vi "UI_page11.vi"(10 "传递队列输入":refnum<queue>, 11 "notifier":refnum<notifier>) -> ()   [LabVIEW 2012]
uses:
  <vilib>/GPower/VIRegister/Library/Convert/ToSGLArry.vi
  <vilib>/GPower/VIRegister/Library/SubVIs/FindRegisterData.vi
  <vilib>/GPower/VIRegister/Library/SubVIs/ReadSub.vi
  <vilib>/GPower/VIRegister/Library/SubVIs/WriteSub.vi
  <vilib>/GPower/VIRegister/Library/QManager/GetRegisterData.vi
  <vilib>/GPower/Error/Library/SetError.vi
  <vilib>/GPower/Error/Library/FilterCodes.vi
  <vilib>/GPower/Error/Library/Filter/FilterMulti.vi
  <vilib>/GPower/VIRegister/Library/QManager/QManagerAction.vi
  <vilib>/GPower/Error/Library/ErrorType.vi
  <vilib>/GPower/Error/Library/SplitAppended.vi
  <vilib>/GPower/Error/Library/SubVIs/ExplanationToError.vi
  <vilib>/GPower/VIRegister/Library/QManager/GetQName.vi
  <vilib>/GPower/VIRegister/Library/QManager/StartQManager.vi
  <vilib>/Utility/error.llb/Trim Whitespace.vi
  <vilib>/dlg_ctls.llb/Space Constant.vi
  <vilib>/Utility/error.llb/Error Code Database.vi
  <vilib>/GPower/Error/Library/SubVIs/SetStatus.vi
  <vilib>/GPower/Error/Library/AppendErrors.vi
  <vilib>/GPower/Error/Library/Append/AppendSingle.vi
  <vilib>/GPower/VIRegister/VIRegister.lvlib
panel:
  in  "主份温控原状态":bool
  in  "备份复位":bool
  in  "主份加计3断电":bool
  in  "主份加计3加电":bool
  in  "主份陀螺3断电":bool
  in  "主份陀螺3加电":bool
  in  "主份温控关闭":bool
  in  "主份加计2断电":bool
  in  "主份加计1断电":bool
  in  "主份加计2加电":bool
  in  "主份加计1加电":bool
  in  "主份陀螺2断电":bool
  in  "主份陀螺1断电":bool
  in  "主份陀螺2加电":bool
  in  "主份陀螺1加电":bool
  in  "主份温控开启":bool
  in  "备份温控原状态":bool
  in  "主份复位":bool
  in  "备份加计3断电":bool
  in  "备份加计3加电":bool
  in  "备份陀螺3断电":bool
  in  "备份陀螺3加电":bool
  in  "备份温控关闭":bool
  in  "备份加计2断电":bool
  in  "备份加计1断电":bool
  in  "备份加计2加电":bool
  in  "备份加计1加电":bool
  in  "备份陀螺2断电":bool
  in  "备份陀螺1断电":bool
  in  "备份陀螺2加电":bool
  in  "备份陀螺1加电":bool
  in  "备份温控开启":bool
  in  "备份切小量程IF电路":bool
  in  "备份切大量程IF电路":bool
  in  "备份加计全断电":bool
  in  "备份加计全加电":bool
  in  "主份切小量程IF电路":bool
  in  "主份切大量程IF电路":bool
  in  "主份加计全断电":bool
  in  "主份加计全加电":bool
  out "模拟量显示区":string
  out "备份自检状态及船舱标志":string
  out "主份自检状态及船舱标志":string
  out "接收数据统计区域":string
  in  "备份复位远程终端":bool
  in  "备份取消发送器关闭":bool
  in  "备份发送器关闭":bool
  in  "备份发送上一状态字":bool
  in  "主份复位远程终端":bool
  in  "主份取消发送器关闭":bool
  in  "主份发送器关闭":bool
  in  "主份发送上一状态字":bool
  in  "备份RT地址选择":enum32{"RT31", "RT21", "RT9"}(radio)
  in  "主份RT地址选择":enum32{"RT31", "RT21", "RT9"}(radio)
  in  "备份通道选择":enum32{"通道A", "通道B"}(radio)
  in  "主份通道选择":enum32{"通道A", "通道B"}(radio)
  in  "备份自定义周期":u16=10 caption="ms" min=10 max=480
  in  "备份周期设置":enum32{"160ms", "自定义", "480ms", "10ms"}(radio)=enum."10ms"
  in  "主份自定义周期":u16=10 caption="ms" min=10 max=480
  in  "主份周期设置":enum32{"160ms", "自定义", "480ms", "10ms"}(radio)=enum."10ms"
  in  "设置存储信息":bool
  in  "备份存储":bool
  in  "主份存储":bool
  # "主份模式指令"
  # "测量存储区"
  # "备份模式指令"
  # "主份指令"
  # "备份指令"
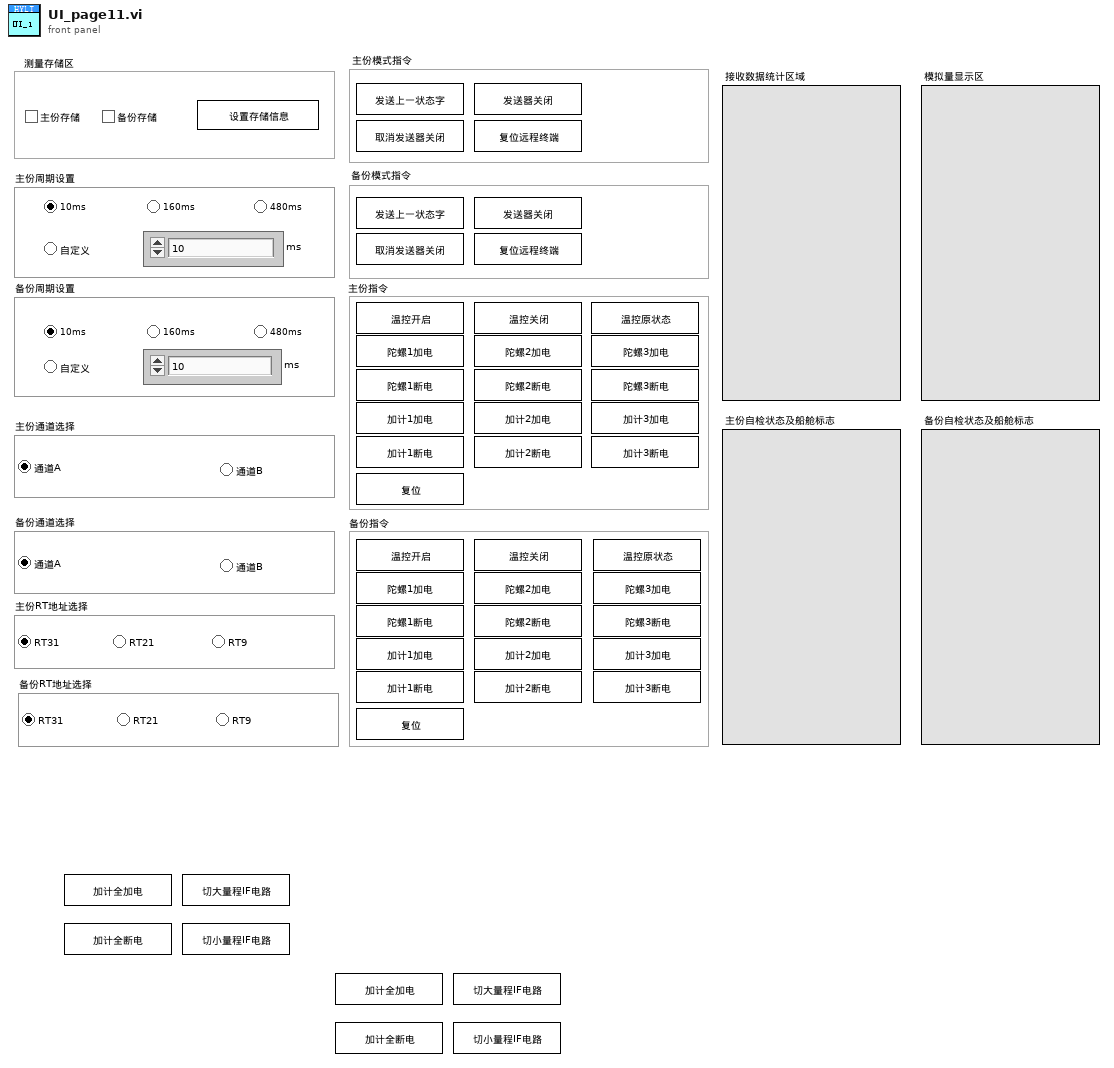
[diagram p1: front panel]
types:
  T1 = cluster{"主份通道选择":enum32{"通道A", "通道B"}, "备份通道选择":enum32{"通道A", "通道B"}}
  T2 = enum32{"invalid app kind", "Development System", "Run Time System", "Student Edition", "Embedded LabVIEW", "Evaluation", "Custom"}
  T3 = enum32{"Invalid", "Standard", "Closed", "Hidden", "Minimized", "Maximized"}
  T4 = cluster{"Core":cluster{"Current VI Reference":refnum<vi>, "Close Panel on Exit?":bool}, "传递队列输入":refnum<queue>, "信息帧":cluster{" 数据帧名称":string, " 数据":string, "备用操作符":bool, "起始地址":i32, "读写标志":i32, "长度":i32}, "主份控制指令":u16, "备份控制指令":u16, "notifier ":refnum<notifier>, "秒计数":i64, "起始时间":i64, "定时控制":bool}
  T5 = cluster{" 数据帧名称":string, " 数据":string, "备用操作符":bool, "起始地址":i32, "读写标志":i32, "长度":i32}
  T6 = cluster{"Current VI Reference":refnum<vi>, "Close Panel on Exit?":bool}
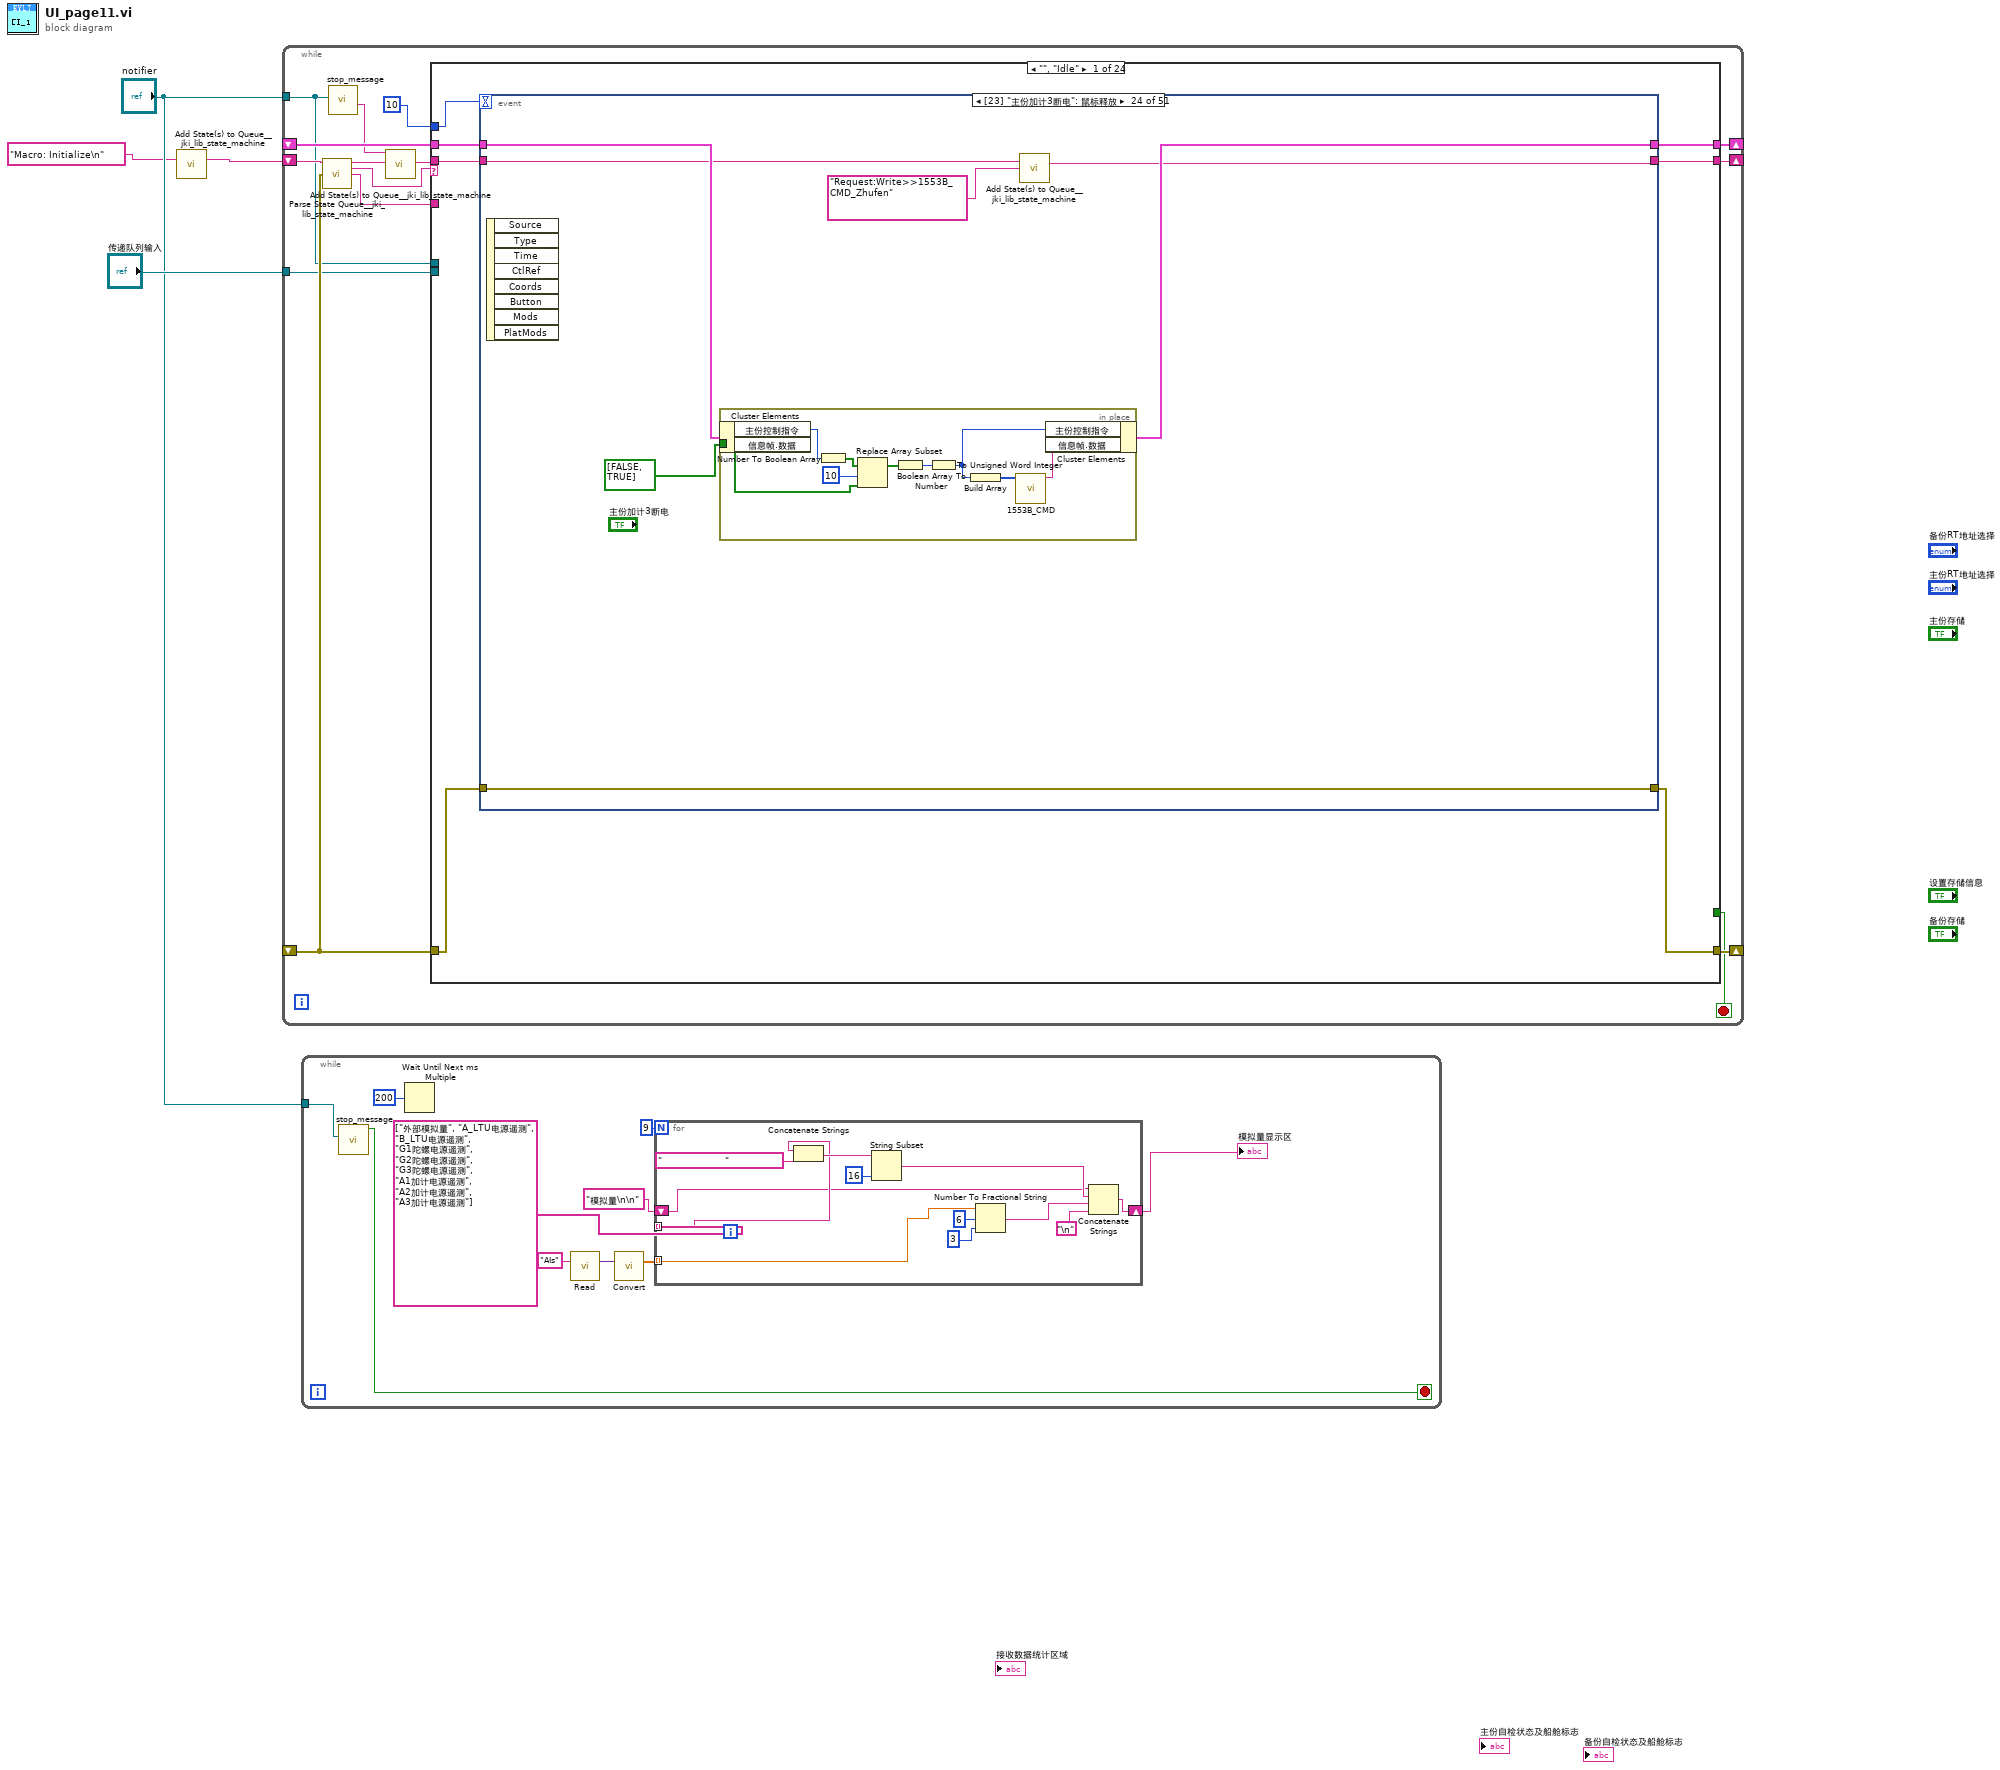
[diagram p0: block diagram]
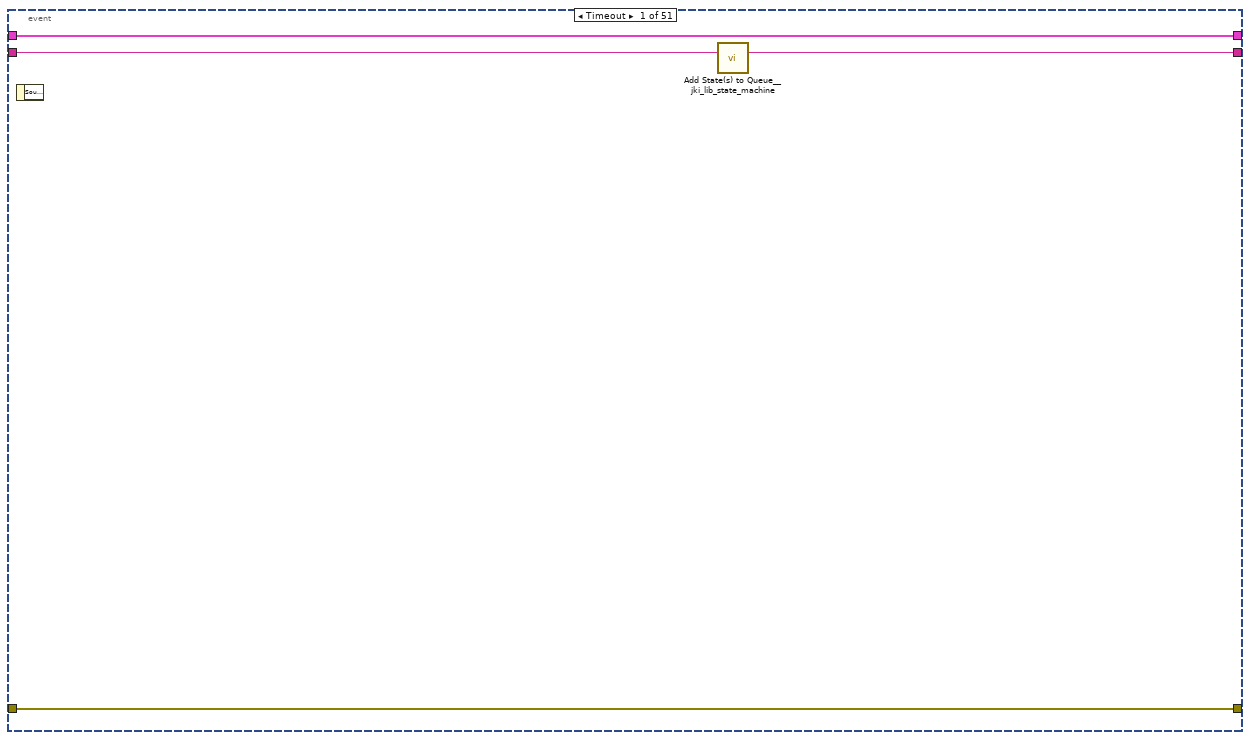
[diagram p2: hidden frame]
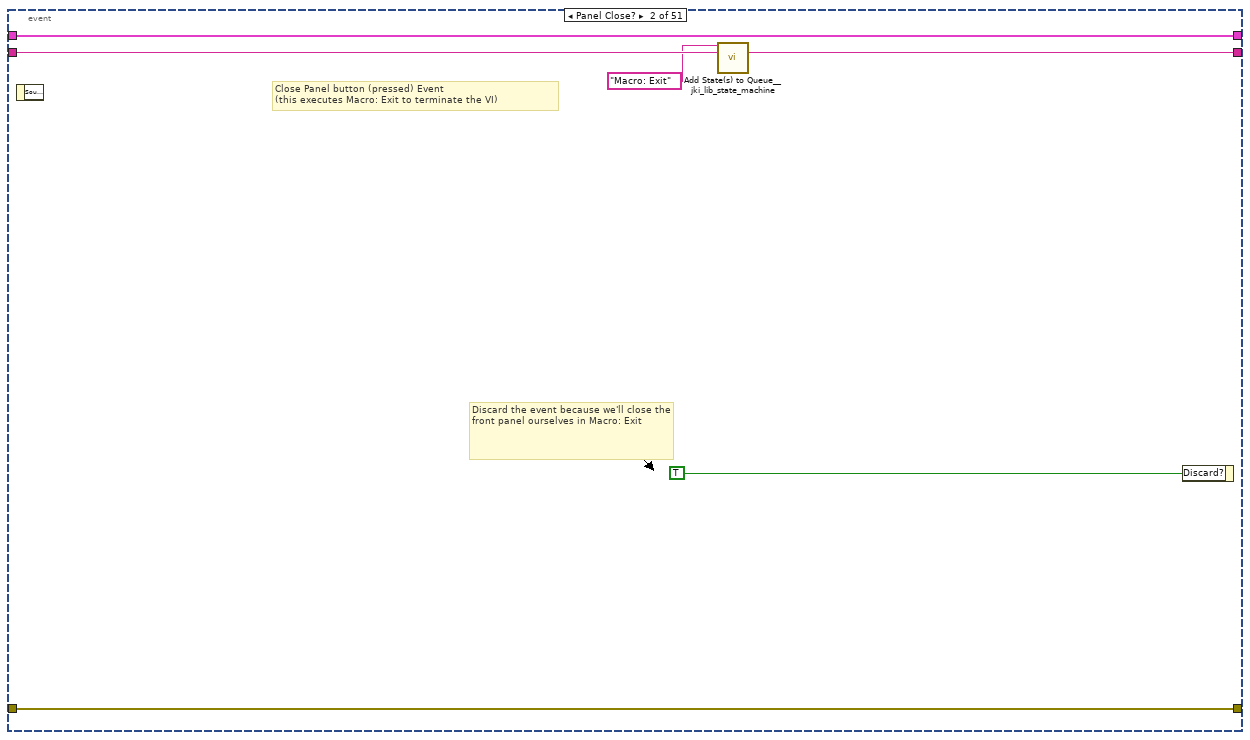
[diagram p3: hidden frame]
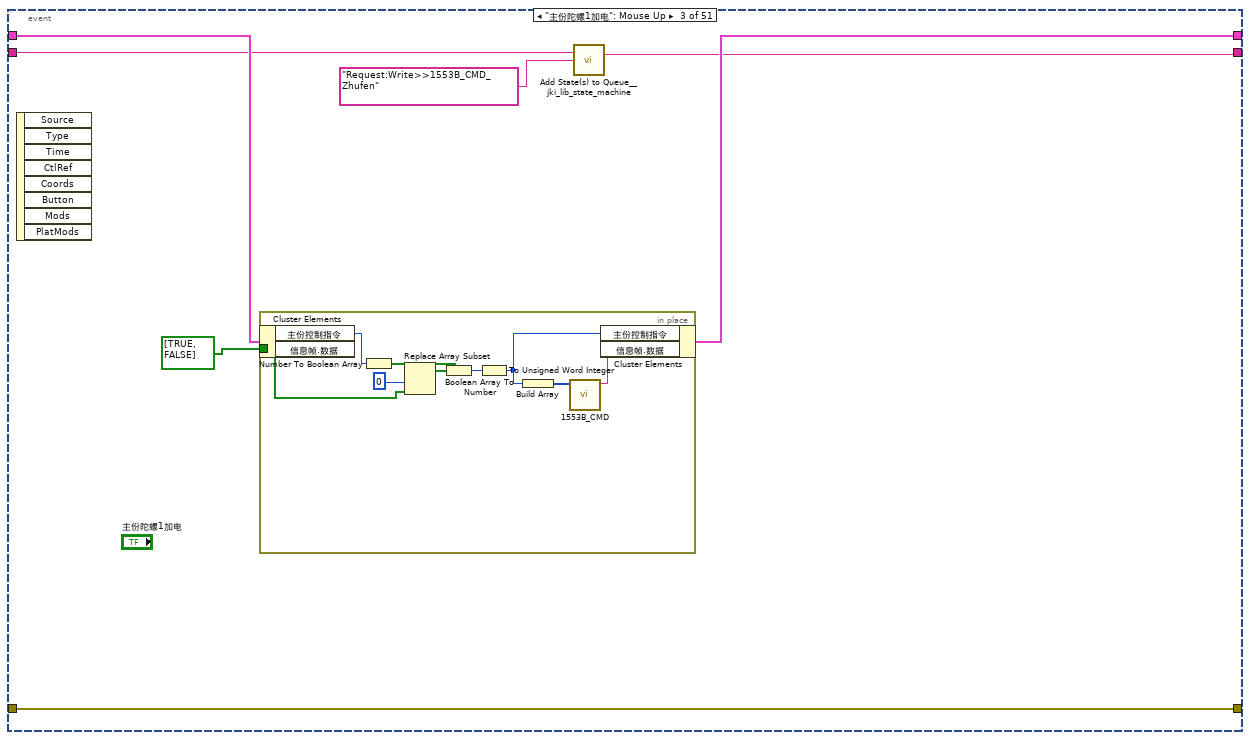
[diagram p4: hidden frame]
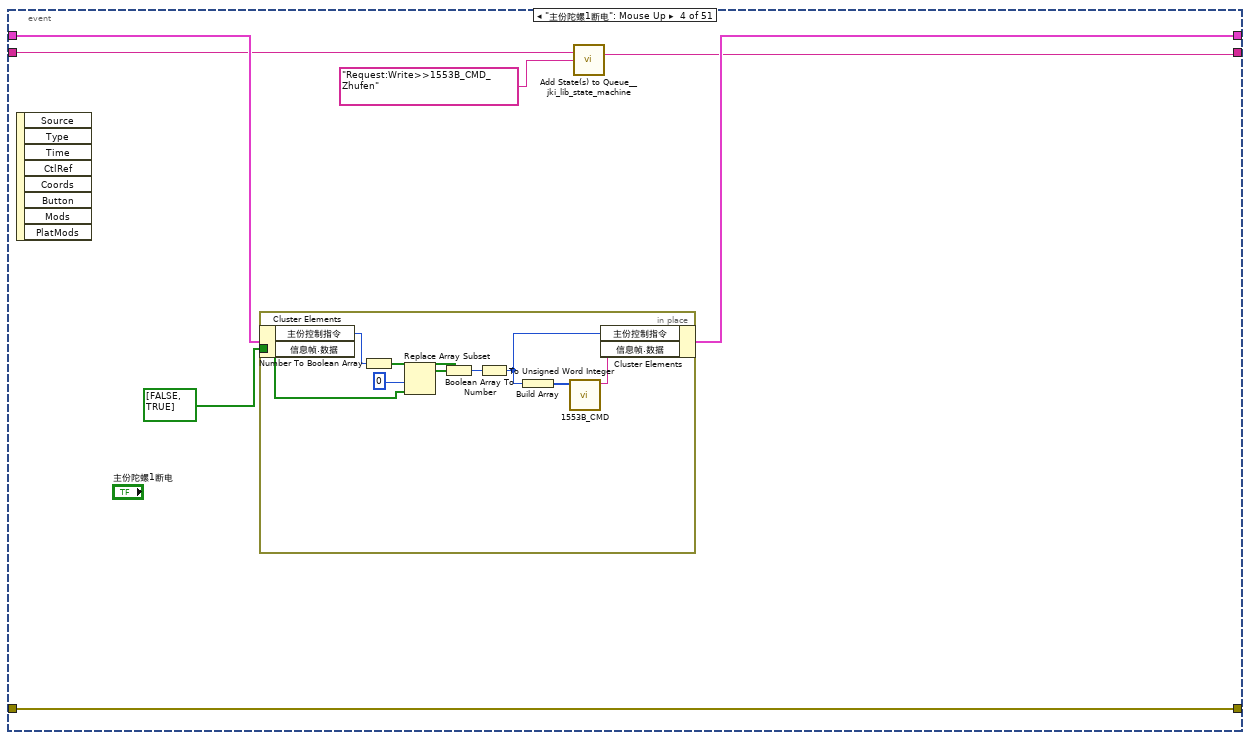
[diagram p5: hidden frame]
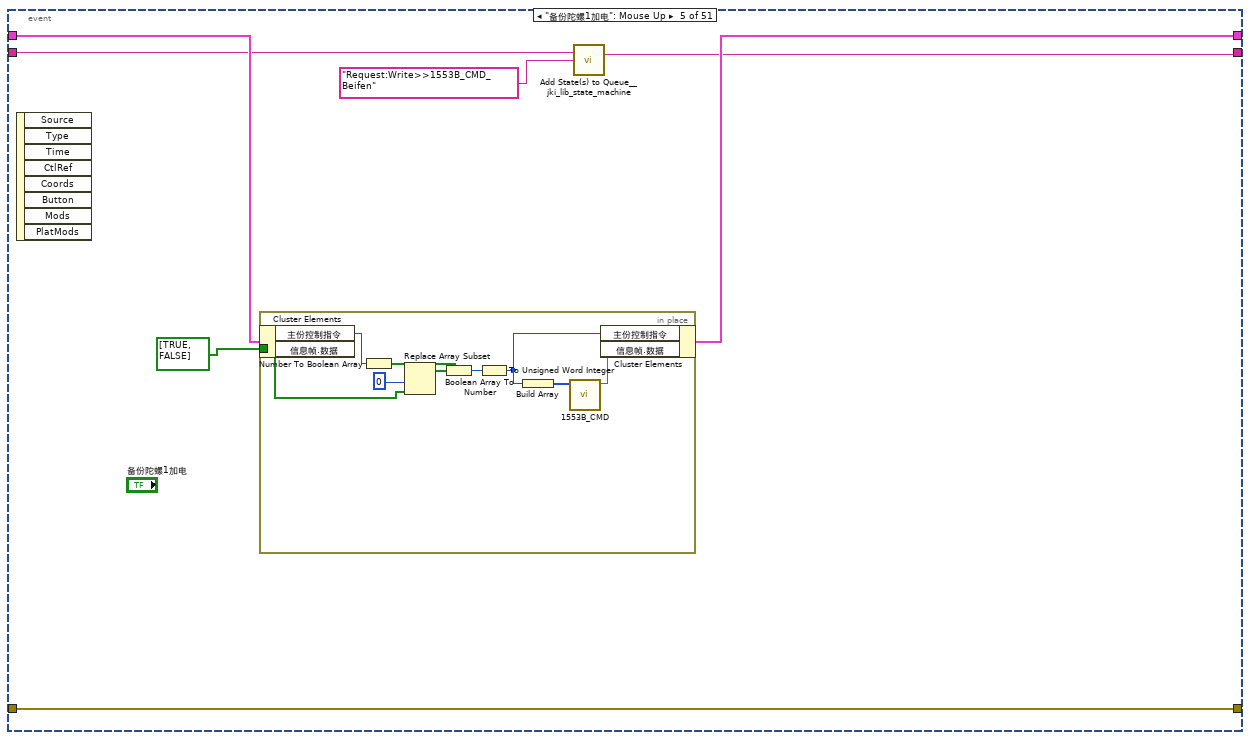
[diagram p6: hidden frame]
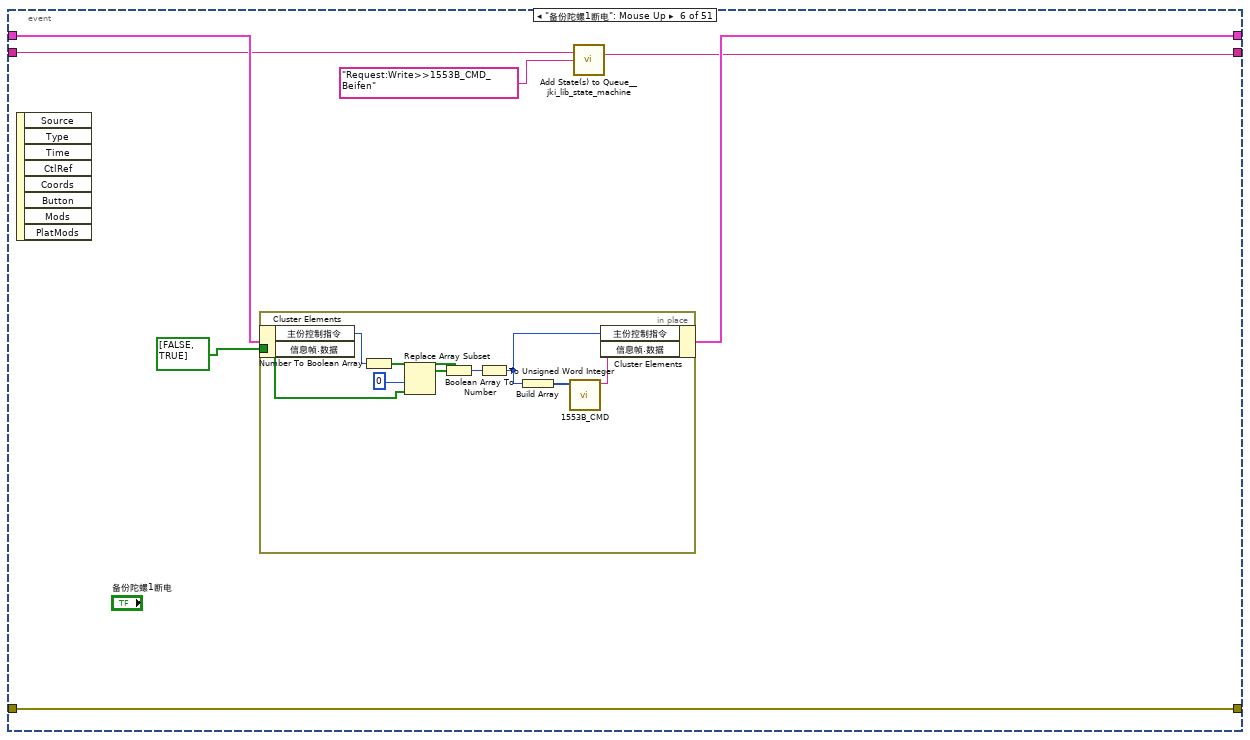
[diagram p7: hidden frame]
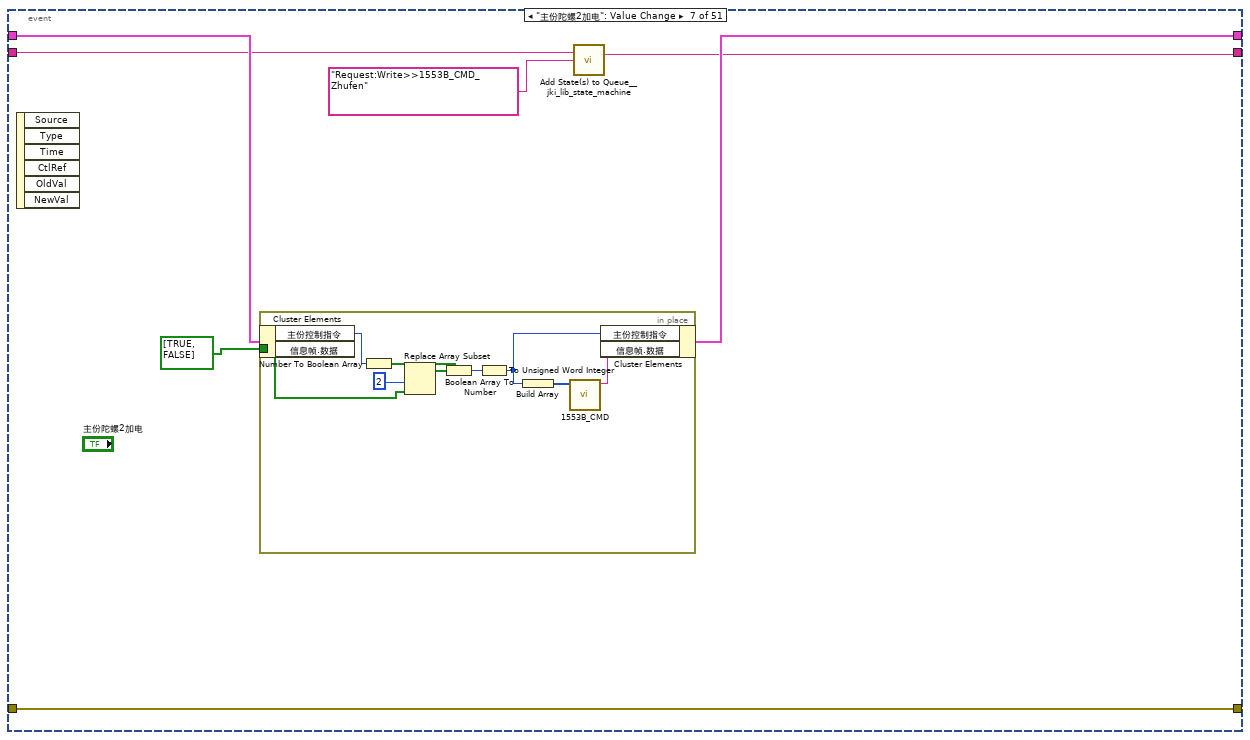
[diagram p8: hidden frame]
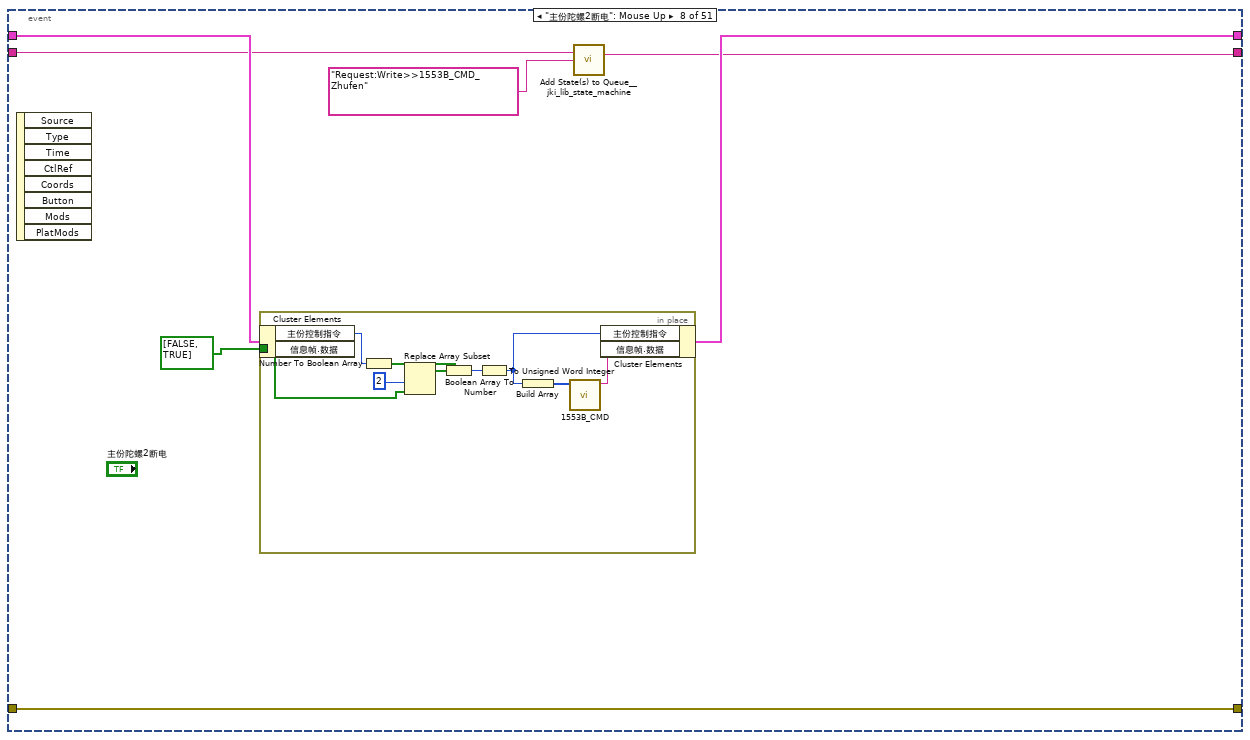
[diagram p9: hidden frame]
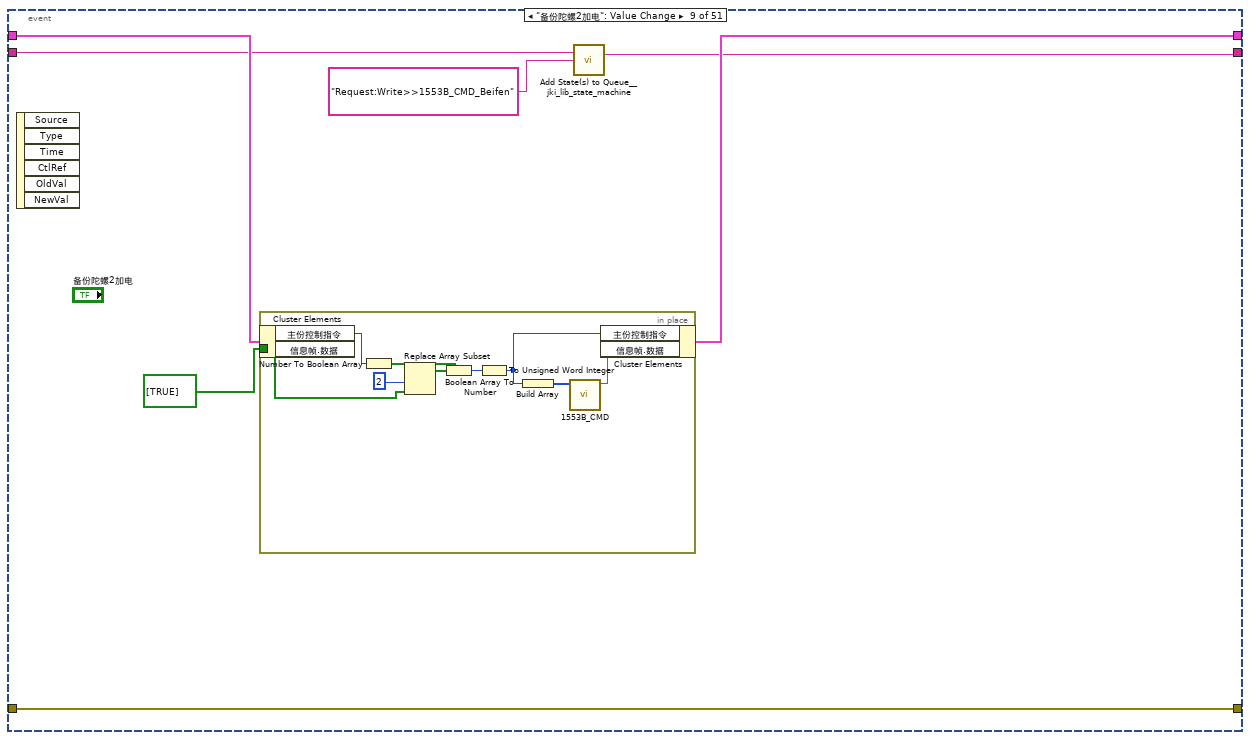
[diagram p10: hidden frame]
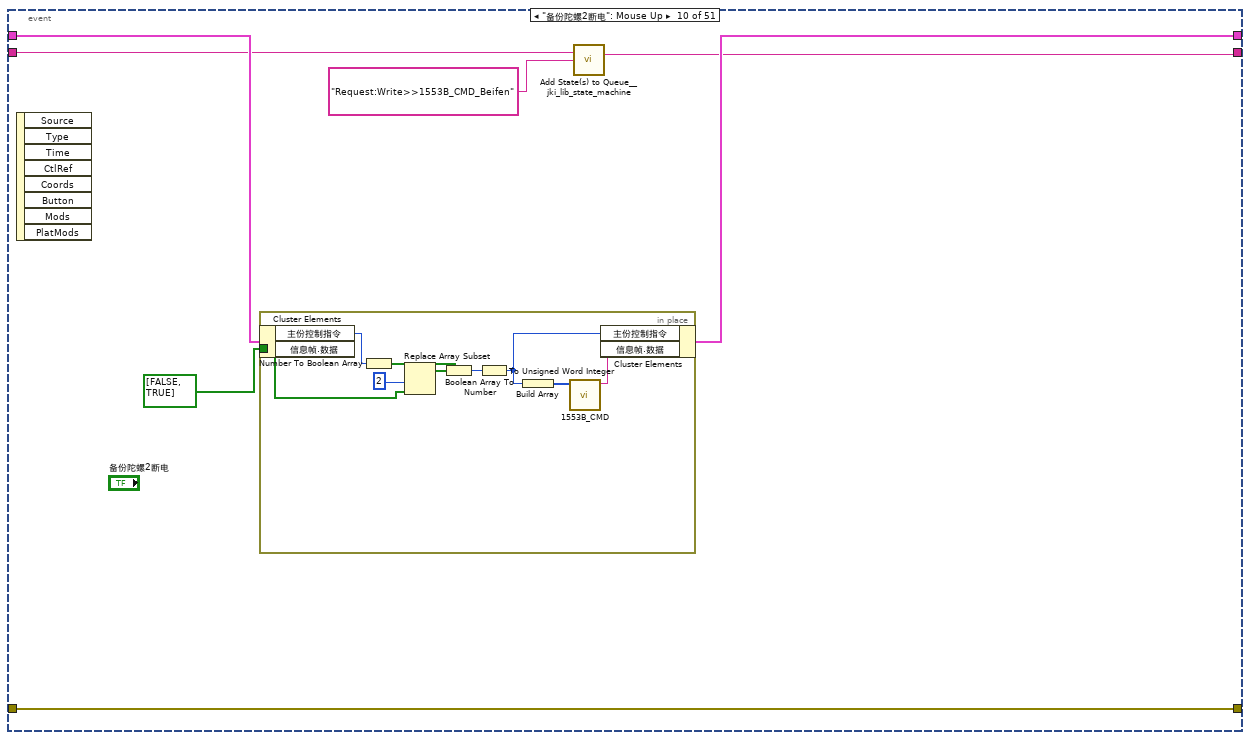
[diagram p11: hidden frame]
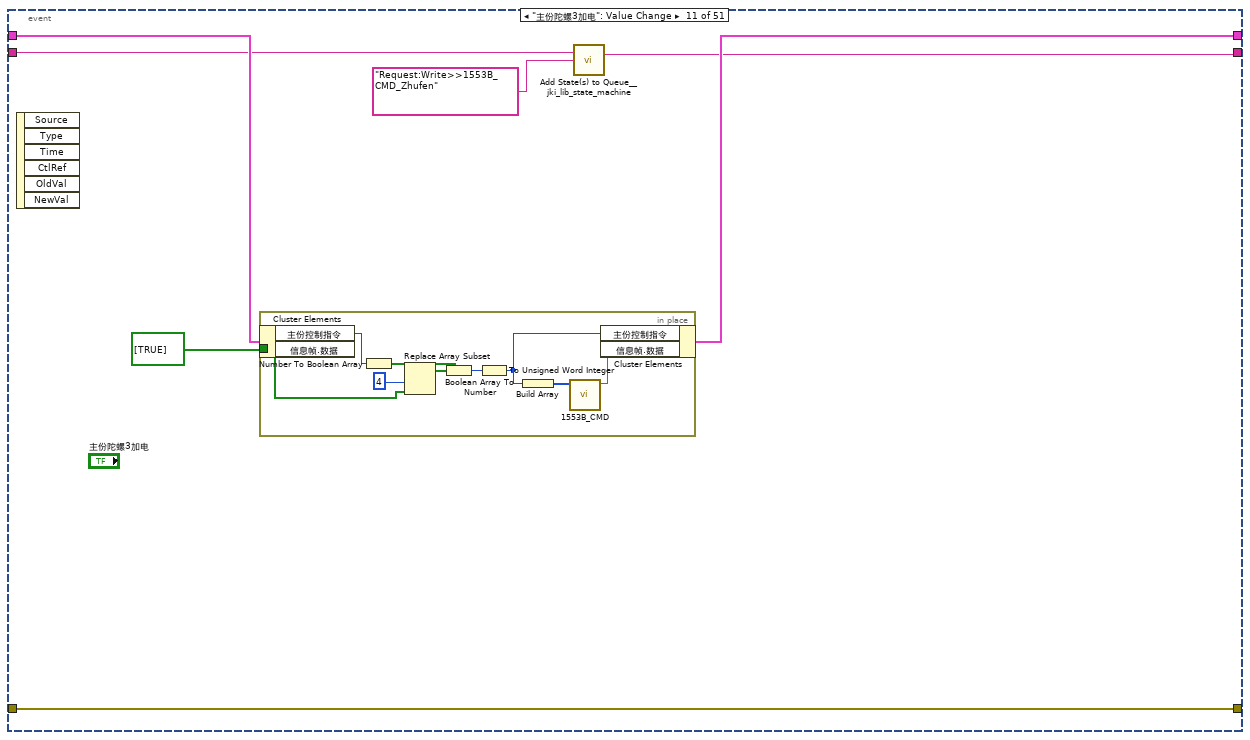
[diagram p12: hidden frame]
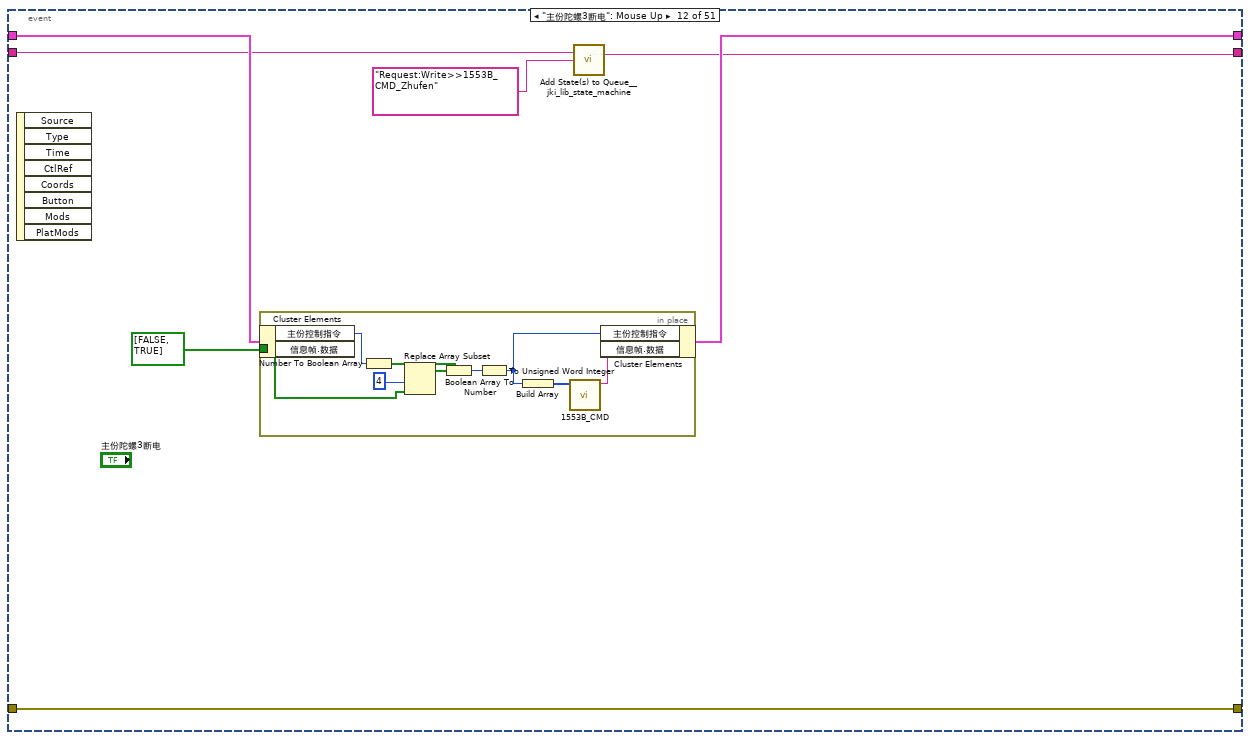
[diagram p13: hidden frame]
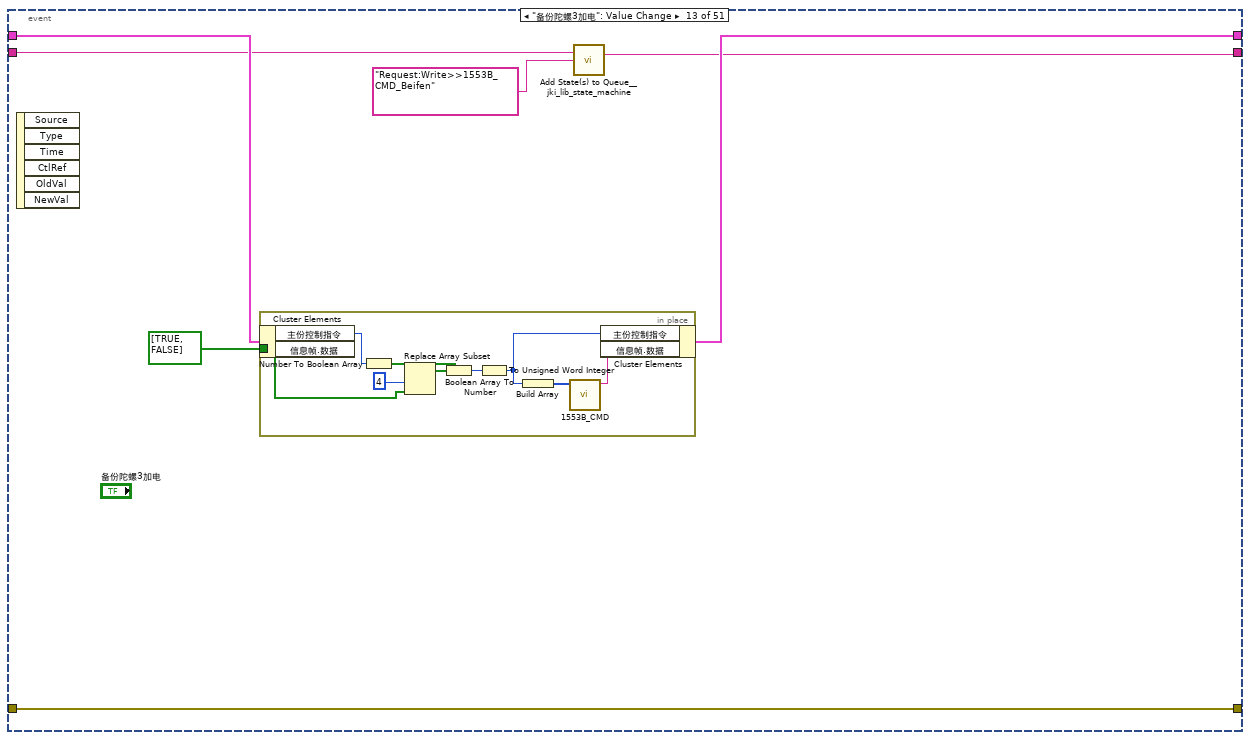
[diagram p14: hidden frame]
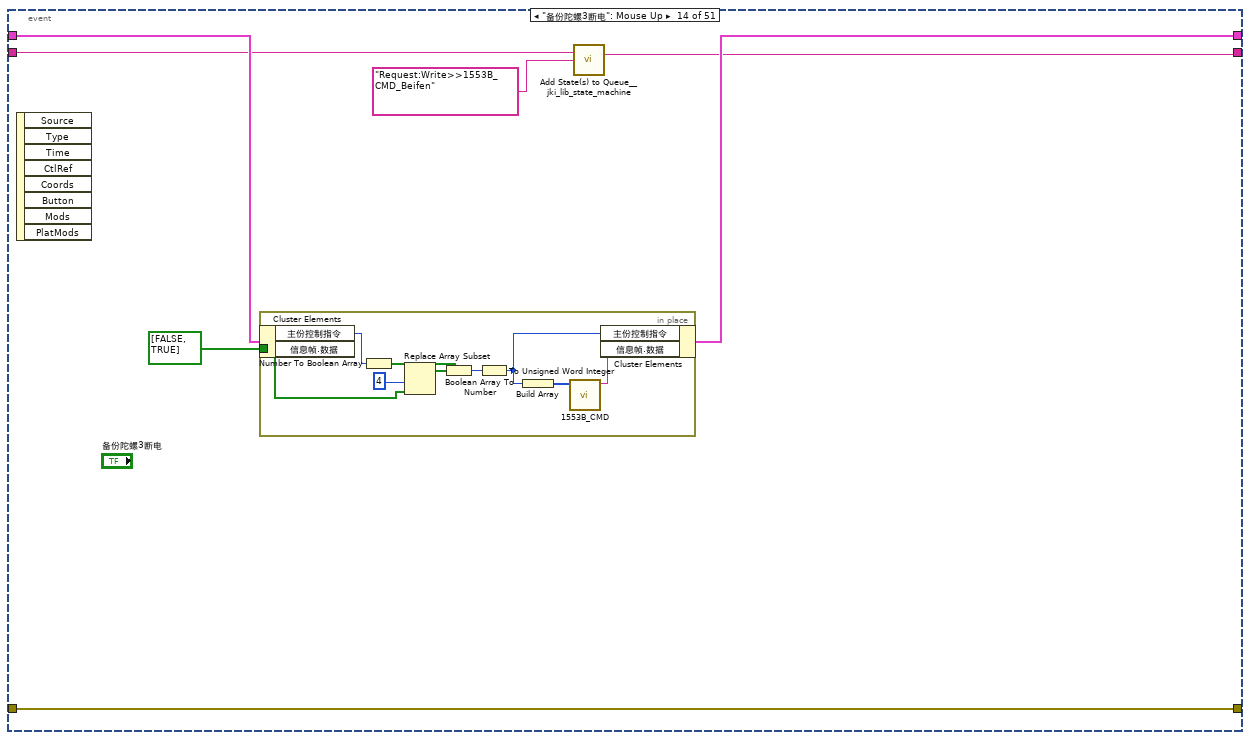
[diagram p15: hidden frame]
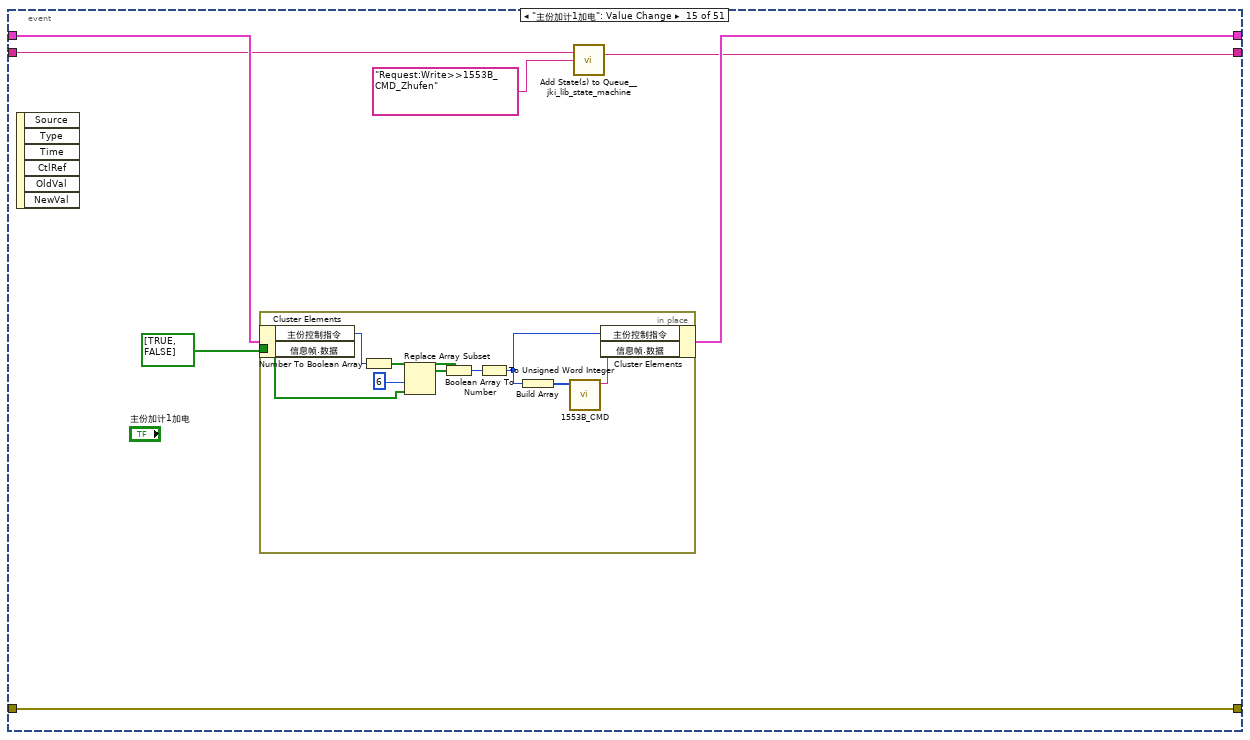
[diagram p16: hidden frame]
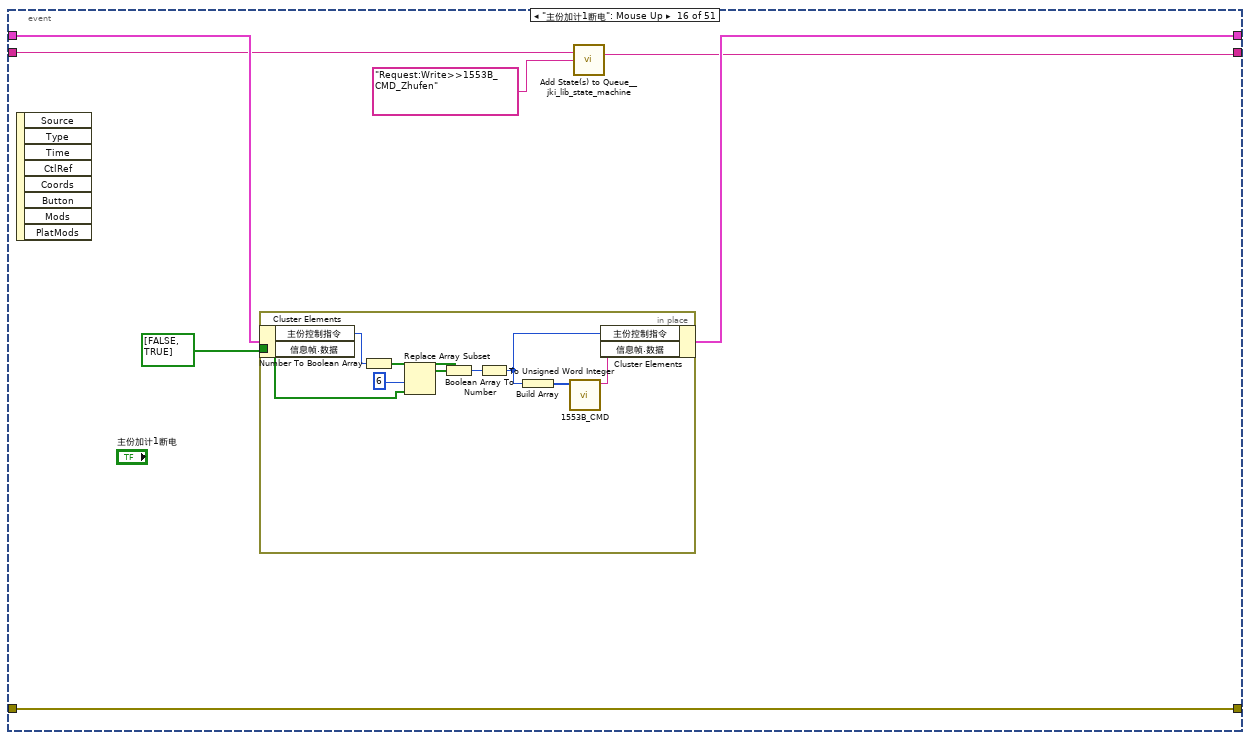
[diagram p17: hidden frame]
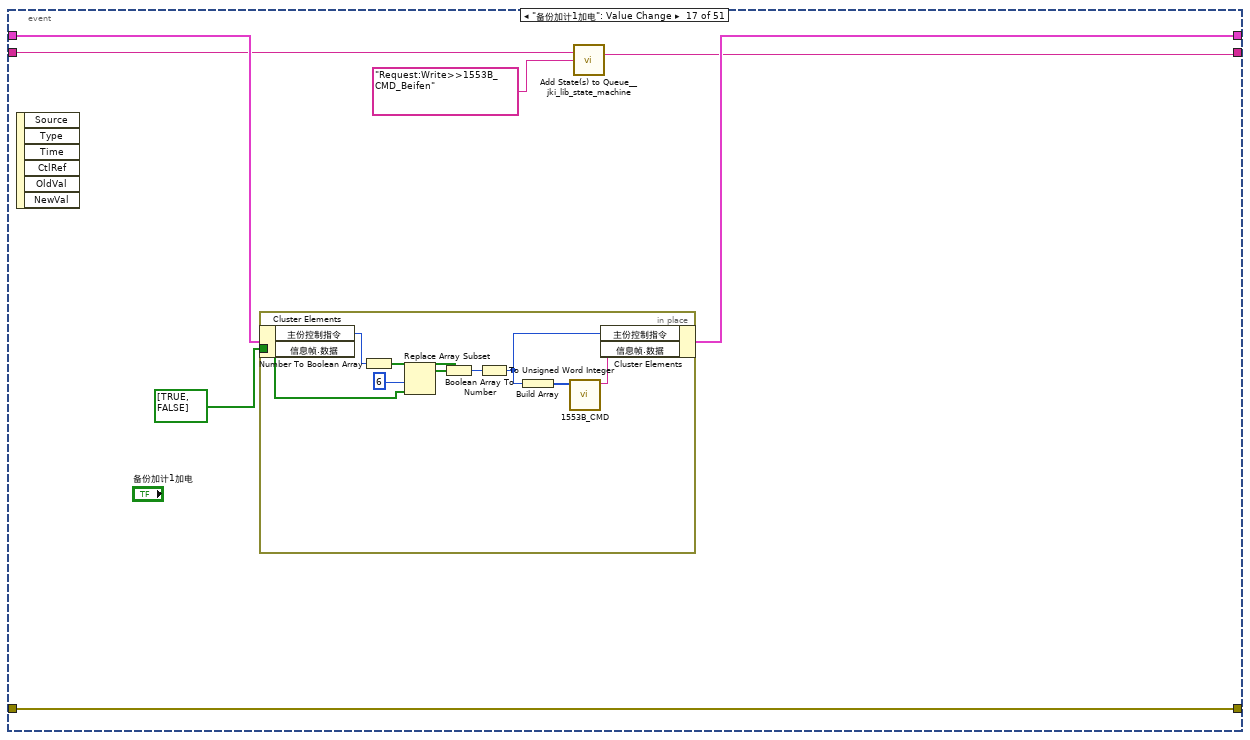
[diagram p18: hidden frame]
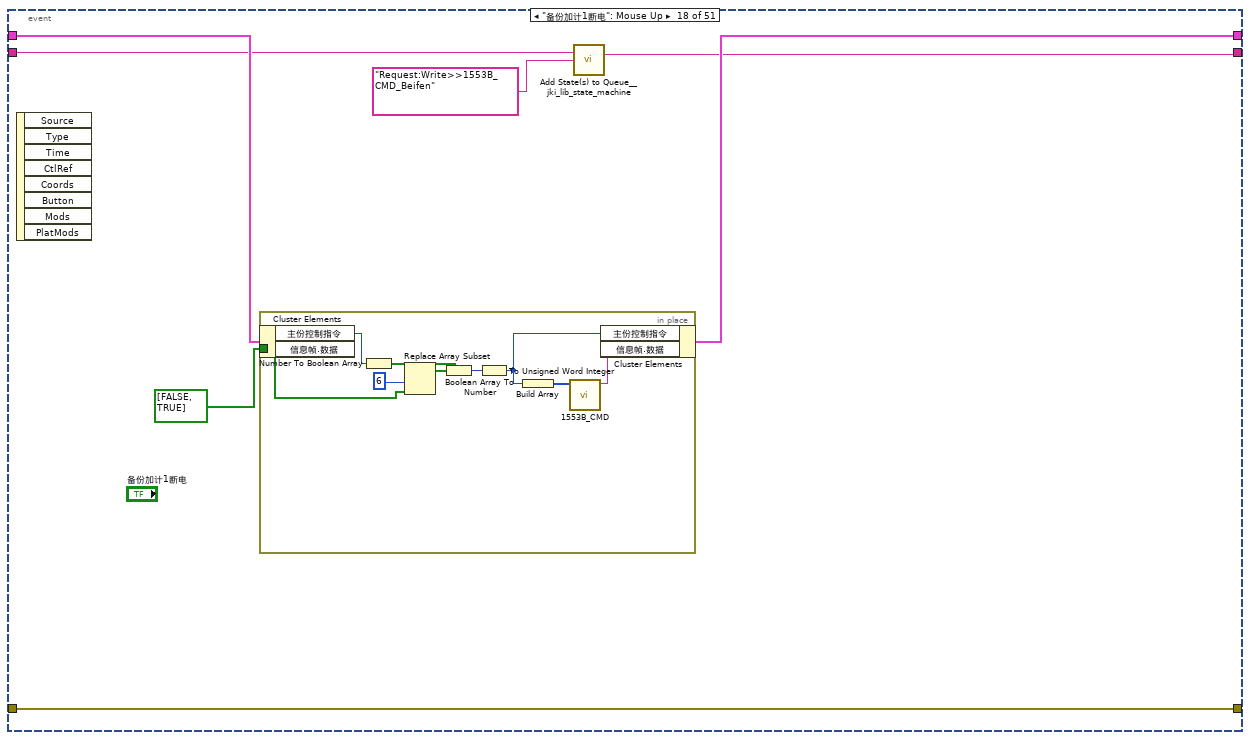
[diagram p19: hidden frame]
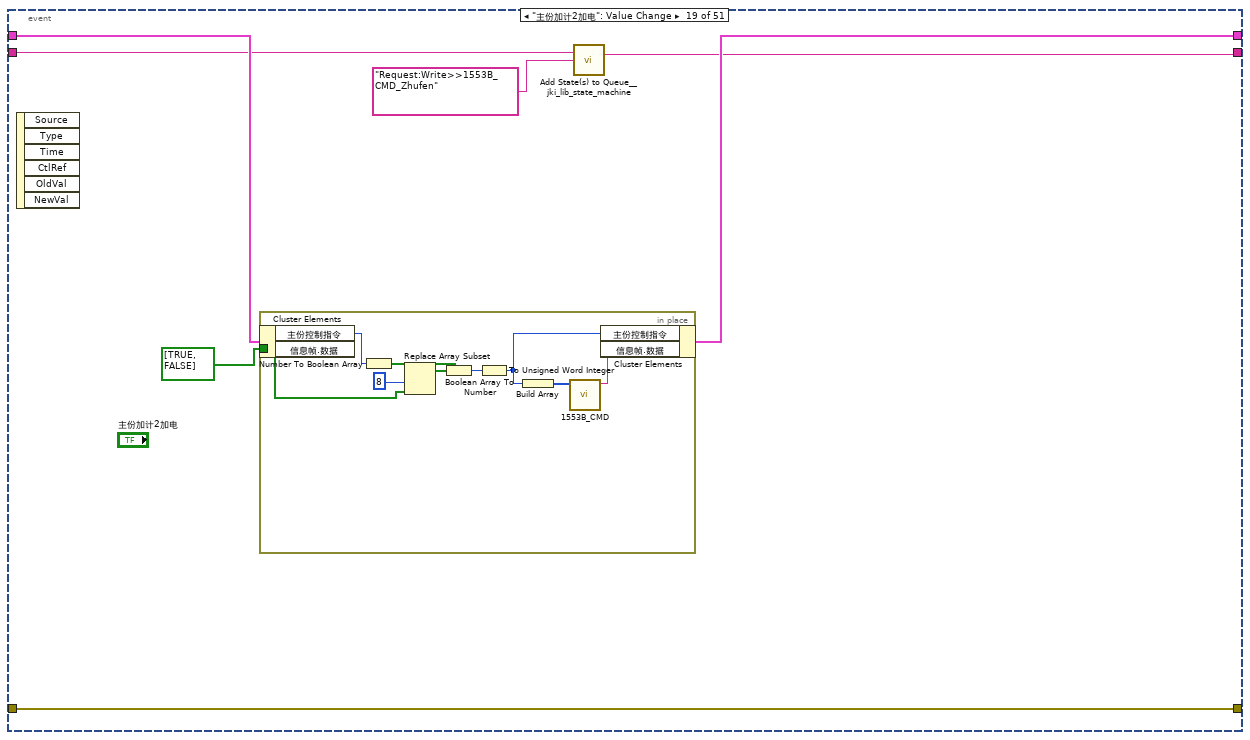
[diagram p20: hidden frame]
diagram:
  n1 = call <vilib>:"Add State(s) to Queue__jki_lib_state_machine.vi"("State(s) in (\"\")"="Macro: Initialize\n") -> ("States Out"=w4:string)  [unwired: 14 in]
  n2 = while "JKI - String-Based Queued State Machine (Basic) v1.0" {
    shift-right: [w13] -> _
    shift-left: _ -> [w12]
    shift-right: [w16] -> _
    shift-left: _ -> [w10]
    shift-right: [w15] -> _
    shift-left: w4 -> [w17]
    tunnel: "notifier" -> [w5]
    tunnel: "传递队列输入" -> [w6]
    stop <- w14 stop-if-true
    n3 = call <vilib>:"Parse State Queue__jki_lib_state_machine.vi"("State Queue"=w17, "Error In (no error)"=w10) -> ("Remaining States"=w9:string, "Current State"=w19:string, "Arguments"=w18:string)  [unwired: 11 in]
    n4 = call "stop_message.vi"("notifier"=w5) -> ("通知"=w8:string)  [unwired: 9 in, 1 out]
    n5 = call <vilib>:"Add State(s) to Queue__jki_lib_state_machine.vi"("State(s) in Front (\"\")"=w8, "State(s) in (\"\")"=w9) -> ("States Out"=w7:string)  [unwired: 13 in]
    n6 = case shown="\"\", \"Idle\"" w19 {
      selector: w19 -> [_ _ w742 _ _ _ _ _ _ _ _ _ _ _ _ _ _ _ _ _ _ _ _ _]
      tunnel: w7 -> [w20 w741 w746 w764 w770 w775 w779 w792 w798 w802 w808 w814 w824 w856 w861 w871 w875 w882 w903 w923 w942 w968 w984 w989]
      tunnel: w18 -> [_ _ _ _ _ _ _ _ _ _ _ w809 w819 _ _ _ _ w876 w897 w917 _ _ _ _]
      tunnel: w12 -> [w25 w738 w744 w755 w767 w773 w776 _ w793 w799 w806 w812 w820 w853 w858 w868 w872 w880 w901 w921 w940 w966 w981 w986]
      tunnel: [w24 w739 w748 w761 errorcluster {"status"=FALSE, "code"=0, "source"=""} ("error out") w772 w777 w789 w794 w800 w805 w810 w821 w854 w859 w869 w873 w878 w899 w919 w938 w964 w982 w987] -> w16
      tunnel: w10 -> [w23 w739 w747 w761 w766 w772 w777 w789 w795 w800 w805 w811 w822 w854 w859 w869 w873 w879 w900 w920 w939 w965 w982 w987]
      tunnel: [w26 w740 w745 w763 w769 w774 w778 w791 w797 w801 w807 w813 w823 w855 w860 w870 w874 w881 w902 w922 w941 w967 w983 w988] -> w15
      tunnel: [_ _ _ _ _ TRUE _ _ _ _ _ _ _ _ _ _ _ _ _ _ _ _ _ _] -> w14
      tunnel: [w22 w738 w744 w762 w767 w773 w776 w790 w793 w799 w806 w812 w820 w853 w858 w868 w872 w877 w898 w918 w937 w963 w981 w986] -> w13
      tunnel: 10 ("Timeout") -> [w21 _ _ _ _ _ _ _ _ _ _ _ _ _ _ _ _ _ _ _ _ _ _ _]
      tunnel: w6 -> [_ _ _ _ _ _ _ w786 _ _ _ _ _ _ _ _ _ _ _ _ _ _ _ _]
      tunnel: w5 -> [_ _ _ _ _ _ _ w783 _ _ _ _ _ _ _ _ _ _ _ _ _ _ _ _]
      frame "", "Idle" {
        n7 = event shown="[23] \"主份加计3断电\": 鼠标释放" {
          selector: _ -> [_ _ _ _ _ _ _ _ _ _ _ _ _ _ _ _ _ _ _ _ _ _ _ _ _ _ _ _ _ _ _ _ _ _ _ _ _ _ _ _ _ _ _ _ _ _ _ _ _ _ _]
          dyn-events: _ -> [_ _ _ _ _ _ _ _ _ _ _ _ _ _ _ _ _ _ _ _ _ _ _ _ _ _ _ _ _ _ _ _ _ _ _ _ _ _ _ _ _ _ _ _ _ _ _ _ _ _ _]
          timeout: w21 -> [_ _ _ _ _ _ _ _ _ _ _ _ _ _ _ _ _ _ _ _ _ _ _ _ _ _ _ _ _ _ _ _ _ _ _ _ _ _ _ _ _ _ _ _ _ _ _ _ _ _ _]
          tunnel: w20 -> [w30 w36 w41 w57 w73 w89 w105 w121 w137 w153 w169 w185 w201 w217 w233 w249 w265 w281 w297 w313 w329 w345 w361 w377 w393 w409 w430 w446 w455 w464 w473 w482 w491 w500 w509 w516 w543 w564 w585 w605 w616 w630 w651 w669 w678 w687 w696 w705 w714 w723 w732]
          tunnel: [w29 w35 w39 w55 w71 w87 w103 w119 w135 w151 w167 w183 w199 w215 w231 w247 w263 w279 w295 w311 w327 w343 w359 w375 w391 w407 w428 w444 w453 w462 w471 w480 w489 w498 w507 w515 w542 w563 w584 w604 w614 w628 w649 w667 w676 w685 w694 w703 w712 w721 w730] -> w26
          tunnel: w25 -> [w27 w33 w43 w59 w75 w91 w107 w123 w139 w155 w171 w187 w203 w219 w235 w251 w267 w283 w299 w315 w331 w347 w363 w379 w395 w411 w422 w448 w457 w466 w475 w484 w493 w502 w511 w518 w546 w566 w587 w602 w618 w632 w653 w671 w680 w689 w698 w707 w716 w725 w734]
          tunnel: [w28 w34 w38 w54 w70 w86 w102 w118 w134 w150 w166 w182 w198 w214 w230 w246 w262 w278 w294 w310 w326 w342 w358 w374 w390 w406 w427 w443 w452 w461 w470 w479 w488 w497 w506 w514 w541 w555 w576 w597 w613 w627 w648 w666 w675 w684 w693 w702 w711 w720 w729] -> w24
          tunnel: w23 -> [w28 w34 w38 w54 w70 w86 w102 w118 w134 w150 w166 w182 w198 w214 w230 w246 w262 w278 w294 w310 w326 w342 w358 w374 w390 w406 w427 w443 w452 w461 w470 w479 w488 w497 w506 w514 w541 w559 w579 w598 w613 w627 w648 w666 w675 w684 w693 w702 w711 w720 w729]
          tunnel: [w27 w33 w42 w58 w74 w90 w106 w122 w138 w154 w170 w186 w202 w218 w234 w250 w266 w282 w298 w314 w330 w346 w362 w378 w394 w410 w421 w447 w456 w465 w474 w483 w492 w501 w510 w517 w544 w565 w586 w601 w617 w631 w652 w670 w679 w688 w697 w706 w715 w724 w733] -> w22
          event Timeout {
            n8 = event-data() -> ()  [unwired: 1 in, 1 out]
            n9 = call <vilib>:"Add State(s) to Queue__jki_lib_state_machine.vi"("State(s) in (\"\")"=w30) -> ("States Out"=w29:string)  [unwired: 14 in]
          }
          event Panel Close? {
            # "Discard the event because we'll close the front panel ourselves in Macro: Exit"
            # "Close Panel button (pressed) Event\n(this executes Macro: Exit to terminate the VI)"
            n10 = event-data() -> ()  [unwired: 1 in, 1 out]
            n11 = call <vilib>:"Add State(s) to Queue__jki_lib_state_machine.vi"("State(s) in Front (\"\")"="Macro: Exit", "State(s) in (\"\")"=w36) -> ("States Out"=w35:string)  [unwired: 13 in]
            n12 = event-data("Discard?"=TRUE) -> ()  [unwired: 1 in, 1 out]
          }
          event "主份陀螺1加电": Mouse Up {
            n13 = event-data() -> ()  [unwired: 1 in, 8 out]
            n14 = in-place {
              in-place-border: bool[] [TRUE, FALSE] -> [w47]
              n15 = in-place-cluster #1(w43) -> ("主份控制指令"=w52:u16)  [unwired: 1 out]
              n16 = Number To Boolean Array(number=w52) -> (Boolean array=w50:bool[])
              n17 = Replace Array Subset(array=w50, new element=w47, index=0 ("索引")) -> (w48:bool[])
              n18 = Boolean Array To Number(Boolean array=w48) -> (number=w51:u32)
              n19 = To Unsigned Word Integer(number=w51) -> (unsigned 16bit integer=w46:u16)
              n20 = Build Array(w46) -> (w45:u16[])
              n21 = call "1553B_CMD.vi"("数据字数组"=w45) -> ("1553B指令"=w44:string)  [unwired: 10 in]
              n22 = in-place-cluster #1("主份控制指令"=w46, "信息帧.数据"=w44) -> (w42:T4)
            }
            n23 = call <vilib>:"Add State(s) to Queue__jki_lib_state_machine.vi"("State(s) in (\"\")"=w41, "State(s) at Back (\"\")"="Request:Write>>1553B_CMD_Zhufen") -> ("States Out"=w39:string)  [unwired: 13 in]
          }
          event "主份陀螺1断电": Mouse Up {
            n24 = event-data() -> ()  [unwired: 1 in, 8 out]
            n25 = in-place {
              in-place-border: bool[] [FALSE, TRUE] -> [w63]
              n26 = in-place-cluster #2(w59) -> ("主份控制指令"=w68:u16)  [unwired: 1 out]
              n27 = Number To Boolean Array(number=w68) -> (Boolean array=w66:bool[])
              n28 = Replace Array Subset(array=w66, new element=w63, index=0 ("索引")) -> (w64:bool[])
              n29 = Boolean Array To Number(Boolean array=w64) -> (number=w67:u32)
              n30 = To Unsigned Word Integer(number=w67) -> (unsigned 16bit integer=w62:u16)
              n31 = Build Array(w62) -> (w61:u16[])
              n32 = call "1553B_CMD.vi"("数据字数组"=w61) -> ("1553B指令"=w60:string)  [unwired: 10 in]
              n33 = in-place-cluster #2("主份控制指令"=w62, "信息帧.数据"=w60) -> (w58:T4)
            }
            n34 = call <vilib>:"Add State(s) to Queue__jki_lib_state_machine.vi"("State(s) in (\"\")"=w57, "State(s) at Back (\"\")"="Request:Write>>1553B_CMD_Zhufen") -> ("States Out"=w55:string)  [unwired: 13 in]
          }
          event "备份陀螺1加电": Mouse Up {
            n35 = event-data() -> ()  [unwired: 1 in, 8 out]
            n36 = in-place {
              in-place-border: bool[] [TRUE, FALSE] -> [w79]
              n37 = in-place-cluster #3(w75) -> ("主份控制指令"=w84:u16)  [unwired: 1 out]
              n38 = Number To Boolean Array(number=w84) -> (Boolean array=w82:bool[])
              n39 = Replace Array Subset(array=w82, new element=w79, index=0 ("索引")) -> (w80:bool[])
              n40 = Boolean Array To Number(Boolean array=w80) -> (number=w83:u32)
              n41 = To Unsigned Word Integer(number=w83) -> (unsigned 16bit integer=w78:u16)
              n42 = Build Array(w78) -> (w77:u16[])
              n43 = call "1553B_CMD.vi"("数据字数组"=w77) -> ("1553B指令"=w76:string)  [unwired: 10 in]
              n44 = in-place-cluster #3("主份控制指令"=w78, "信息帧.数据"=w76) -> (w74:T4)
            }
            n45 = call <vilib>:"Add State(s) to Queue__jki_lib_state_machine.vi"("State(s) in (\"\")"=w73, "State(s) at Back (\"\")"="Request:Write>>1553B_CMD_Beifen") -> ("States Out"=w71:string)  [unwired: 13 in]
          }
          event "备份陀螺1断电": Mouse Up {
            n46 = event-data() -> ()  [unwired: 1 in, 8 out]
            n47 = in-place {
              in-place-border: bool[] [FALSE, TRUE] -> [w95]
              n48 = in-place-cluster #4(w91) -> ("主份控制指令"=w100:u16)  [unwired: 1 out]
              n49 = Number To Boolean Array(number=w100) -> (Boolean array=w98:bool[])
              n50 = Replace Array Subset(array=w98, new element=w95, index=0 ("索引")) -> (w96:bool[])
              n51 = Boolean Array To Number(Boolean array=w96) -> (number=w99:u32)
              n52 = To Unsigned Word Integer(number=w99) -> (unsigned 16bit integer=w94:u16)
              n53 = Build Array(w94) -> (w93:u16[])
              n54 = call "1553B_CMD.vi"("数据字数组"=w93) -> ("1553B指令"=w92:string)  [unwired: 10 in]
              n55 = in-place-cluster #4("主份控制指令"=w94, "信息帧.数据"=w92) -> (w90:T4)
            }
            n56 = call <vilib>:"Add State(s) to Queue__jki_lib_state_machine.vi"("State(s) in (\"\")"=w89, "State(s) at Back (\"\")"="Request:Write>>1553B_CMD_Beifen") -> ("States Out"=w87:string)  [unwired: 13 in]
          }
          event "主份陀螺2加电": Value Change {
            n57 = event-data() -> ()  [unwired: 1 in, 6 out]
            n58 = in-place {
              in-place-border: bool[] [TRUE, FALSE] -> [w111]
              n59 = in-place-cluster #5(w107) -> ("主份控制指令"=w116:u16)  [unwired: 1 out]
              n60 = Number To Boolean Array(number=w116) -> (Boolean array=w114:bool[])
              n61 = Replace Array Subset(array=w114, new element=w111, index=2 ("索引")) -> (w112:bool[])
              n62 = Boolean Array To Number(Boolean array=w112) -> (number=w115:u32)
              n63 = To Unsigned Word Integer(number=w115) -> (unsigned 16bit integer=w110:u16)
              n64 = Build Array(w110) -> (w109:u16[])
              n65 = call "1553B_CMD.vi"("数据字数组"=w109) -> ("1553B指令"=w108:string)  [unwired: 10 in]
              n66 = in-place-cluster #5("主份控制指令"=w110, "信息帧.数据"=w108) -> (w106:T4)
            }
            n67 = call <vilib>:"Add State(s) to Queue__jki_lib_state_machine.vi"("State(s) in (\"\")"=w105, "State(s) at Back (\"\")"="Request:Write>>1553B_CMD_Zhufen") -> ("States Out"=w103:string)  [unwired: 13 in]
          }
          event "主份陀螺2断电": Mouse Up {
            n68 = event-data() -> ()  [unwired: 1 in, 8 out]
            n69 = in-place {
              in-place-border: bool[] [FALSE, TRUE] -> [w127]
              n70 = in-place-cluster #6(w123) -> ("主份控制指令"=w132:u16)  [unwired: 1 out]
              n71 = Number To Boolean Array(number=w132) -> (Boolean array=w130:bool[])
              n72 = Replace Array Subset(array=w130, new element=w127, index=2 ("索引")) -> (w128:bool[])
              n73 = Boolean Array To Number(Boolean array=w128) -> (number=w131:u32)
              n74 = To Unsigned Word Integer(number=w131) -> (unsigned 16bit integer=w126:u16)
              n75 = Build Array(w126) -> (w125:u16[])
              n76 = call "1553B_CMD.vi"("数据字数组"=w125) -> ("1553B指令"=w124:string)  [unwired: 10 in]
              n77 = in-place-cluster #6("主份控制指令"=w126, "信息帧.数据"=w124) -> (w122:T4)
            }
            n78 = call <vilib>:"Add State(s) to Queue__jki_lib_state_machine.vi"("State(s) in (\"\")"=w121, "State(s) at Back (\"\")"="Request:Write>>1553B_CMD_Zhufen") -> ("States Out"=w119:string)  [unwired: 13 in]
          }
          event "备份陀螺2加电": Value Change {
            n79 = event-data() -> ()  [unwired: 1 in, 6 out]
            n80 = in-place {
              in-place-border: bool[] [TRUE] -> [w143]
              n81 = in-place-cluster #7(w139) -> ("主份控制指令"=w148:u16)  [unwired: 1 out]
              n82 = Number To Boolean Array(number=w148) -> (Boolean array=w146:bool[])
              n83 = Replace Array Subset(array=w146, new element=w143, index=2 ("索引")) -> (w144:bool[])
              n84 = Boolean Array To Number(Boolean array=w144) -> (number=w147:u32)
              n85 = To Unsigned Word Integer(number=w147) -> (unsigned 16bit integer=w142:u16)
              n86 = Build Array(w142) -> (w141:u16[])
              n87 = call "1553B_CMD.vi"("数据字数组"=w141) -> ("1553B指令"=w140:string)  [unwired: 10 in]
              n88 = in-place-cluster #7("主份控制指令"=w142, "信息帧.数据"=w140) -> (w138:T4)
            }
            n89 = call <vilib>:"Add State(s) to Queue__jki_lib_state_machine.vi"("State(s) in (\"\")"=w137, "State(s) at Back (\"\")"="Request:Write>>1553B_CMD_Beifen") -> ("States Out"=w135:string)  [unwired: 13 in]
          }
          event "备份陀螺2断电": Mouse Up {
            n90 = event-data() -> ()  [unwired: 1 in, 8 out]
            n91 = in-place {
              in-place-border: bool[] [FALSE, TRUE] -> [w159]
              n92 = in-place-cluster #8(w155) -> ("主份控制指令"=w164:u16)  [unwired: 1 out]
              n93 = Number To Boolean Array(number=w164) -> (Boolean array=w162:bool[])
              n94 = Replace Array Subset(array=w162, new element=w159, index=2 ("索引")) -> (w160:bool[])
              n95 = Boolean Array To Number(Boolean array=w160) -> (number=w163:u32)
              n96 = To Unsigned Word Integer(number=w163) -> (unsigned 16bit integer=w158:u16)
              n97 = Build Array(w158) -> (w157:u16[])
              n98 = call "1553B_CMD.vi"("数据字数组"=w157) -> ("1553B指令"=w156:string)  [unwired: 10 in]
              n99 = in-place-cluster #8("主份控制指令"=w158, "信息帧.数据"=w156) -> (w154:T4)
            }
            n100 = call <vilib>:"Add State(s) to Queue__jki_lib_state_machine.vi"("State(s) in (\"\")"=w153, "State(s) at Back (\"\")"="Request:Write>>1553B_CMD_Beifen") -> ("States Out"=w151:string)  [unwired: 13 in]
          }
          event "主份陀螺3加电": Value Change {
            n101 = event-data() -> ()  [unwired: 1 in, 6 out]
            n102 = in-place {
              in-place-border: bool[] [TRUE] -> [w175]
              n103 = in-place-cluster #9(w171) -> ("主份控制指令"=w180:u16)  [unwired: 1 out]
              n104 = Number To Boolean Array(number=w180) -> (Boolean array=w178:bool[])
              n105 = Replace Array Subset(array=w178, new element=w175, index=4 ("索引")) -> (w176:bool[])
              n106 = Boolean Array To Number(Boolean array=w176) -> (number=w179:u32)
              n107 = To Unsigned Word Integer(number=w179) -> (unsigned 16bit integer=w174:u16)
              n108 = Build Array(w174) -> (w173:u16[])
              n109 = call "1553B_CMD.vi"("数据字数组"=w173) -> ("1553B指令"=w172:string)  [unwired: 10 in]
              n110 = in-place-cluster #9("主份控制指令"=w174, "信息帧.数据"=w172) -> (w170:T4)
            }
            n111 = call <vilib>:"Add State(s) to Queue__jki_lib_state_machine.vi"("State(s) in (\"\")"=w169, "State(s) at Back (\"\")"="Request:Write>>1553B_CMD_Zhufen") -> ("States Out"=w167:string)  [unwired: 13 in]
          }
          event "主份陀螺3断电": Mouse Up {
            n112 = event-data() -> ()  [unwired: 1 in, 8 out]
            n113 = in-place {
              in-place-border: bool[] [FALSE, TRUE] -> [w191]
              n114 = in-place-cluster #10(w187) -> ("主份控制指令"=w196:u16)  [unwired: 1 out]
              n115 = Number To Boolean Array(number=w196) -> (Boolean array=w194:bool[])
              n116 = Replace Array Subset(array=w194, new element=w191, index=4 ("索引")) -> (w192:bool[])
              n117 = Boolean Array To Number(Boolean array=w192) -> (number=w195:u32)
              n118 = To Unsigned Word Integer(number=w195) -> (unsigned 16bit integer=w190:u16)
              n119 = Build Array(w190) -> (w189:u16[])
              n120 = call "1553B_CMD.vi"("数据字数组"=w189) -> ("1553B指令"=w188:string)  [unwired: 10 in]
              n121 = in-place-cluster #10("主份控制指令"=w190, "信息帧.数据"=w188) -> (w186:T4)
            }
            n122 = call <vilib>:"Add State(s) to Queue__jki_lib_state_machine.vi"("State(s) in (\"\")"=w185, "State(s) at Back (\"\")"="Request:Write>>1553B_CMD_Zhufen") -> ("States Out"=w183:string)  [unwired: 13 in]
          }
          event "备份陀螺3加电": Value Change {
            n123 = event-data() -> ()  [unwired: 1 in, 6 out]
            n124 = in-place {
              in-place-border: bool[] [TRUE, FALSE] -> [w207]
              n125 = in-place-cluster #11(w203) -> ("主份控制指令"=w212:u16)  [unwired: 1 out]
              n126 = Number To Boolean Array(number=w212) -> (Boolean array=w210:bool[])
              n127 = Replace Array Subset(array=w210, new element=w207, index=4 ("索引")) -> (w208:bool[])
              n128 = Boolean Array To Number(Boolean array=w208) -> (number=w211:u32)
              n129 = To Unsigned Word Integer(number=w211) -> (unsigned 16bit integer=w206:u16)
              n130 = Build Array(w206) -> (w205:u16[])
              n131 = call "1553B_CMD.vi"("数据字数组"=w205) -> ("1553B指令"=w204:string)  [unwired: 10 in]
              n132 = in-place-cluster #11("主份控制指令"=w206, "信息帧.数据"=w204) -> (w202:T4)
            }
            n133 = call <vilib>:"Add State(s) to Queue__jki_lib_state_machine.vi"("State(s) in (\"\")"=w201, "State(s) at Back (\"\")"="Request:Write>>1553B_CMD_Beifen") -> ("States Out"=w199:string)  [unwired: 13 in]
          }
          event "备份陀螺3断电": Mouse Up {
            n134 = event-data() -> ()  [unwired: 1 in, 8 out]
            n135 = in-place {
              in-place-border: bool[] [FALSE, TRUE] -> [w223]
              n136 = in-place-cluster #12(w219) -> ("主份控制指令"=w228:u16)  [unwired: 1 out]
              n137 = Number To Boolean Array(number=w228) -> (Boolean array=w226:bool[])
              n138 = Replace Array Subset(array=w226, new element=w223, index=4 ("索引")) -> (w224:bool[])
              n139 = Boolean Array To Number(Boolean array=w224) -> (number=w227:u32)
              n140 = To Unsigned Word Integer(number=w227) -> (unsigned 16bit integer=w222:u16)
              n141 = Build Array(w222) -> (w221:u16[])
              n142 = call "1553B_CMD.vi"("数据字数组"=w221) -> ("1553B指令"=w220:string)  [unwired: 10 in]
              n143 = in-place-cluster #12("主份控制指令"=w222, "信息帧.数据"=w220) -> (w218:T4)
            }
            n144 = call <vilib>:"Add State(s) to Queue__jki_lib_state_machine.vi"("State(s) in (\"\")"=w217, "State(s) at Back (\"\")"="Request:Write>>1553B_CMD_Beifen") -> ("States Out"=w215:string)  [unwired: 13 in]
          }
          event "主份加计1加电": Value Change {
            n145 = event-data() -> ()  [unwired: 1 in, 6 out]
            n146 = in-place {
              in-place-border: bool[] [TRUE, FALSE] -> [w239]
              n147 = in-place-cluster #13(w235) -> ("主份控制指令"=w244:u16)  [unwired: 1 out]
              n148 = Number To Boolean Array(number=w244) -> (Boolean array=w242:bool[])
              n149 = Replace Array Subset(array=w242, new element=w239, index=6 ("索引")) -> (w240:bool[])
              n150 = Boolean Array To Number(Boolean array=w240) -> (number=w243:u32)
              n151 = To Unsigned Word Integer(number=w243) -> (unsigned 16bit integer=w238:u16)
              n152 = Build Array(w238) -> (w237:u16[])
              n153 = call "1553B_CMD.vi"("数据字数组"=w237) -> ("1553B指令"=w236:string)  [unwired: 10 in]
              n154 = in-place-cluster #13("主份控制指令"=w238, "信息帧.数据"=w236) -> (w234:T4)
            }
            n155 = call <vilib>:"Add State(s) to Queue__jki_lib_state_machine.vi"("State(s) in (\"\")"=w233, "State(s) at Back (\"\")"="Request:Write>>1553B_CMD_Zhufen") -> ("States Out"=w231:string)  [unwired: 13 in]
          }
          event "主份加计1断电": Mouse Up {
            n156 = event-data() -> ()  [unwired: 1 in, 8 out]
            n157 = in-place {
              in-place-border: bool[] [FALSE, TRUE] -> [w255]
              n158 = in-place-cluster #14(w251) -> ("主份控制指令"=w260:u16)  [unwired: 1 out]
              n159 = Number To Boolean Array(number=w260) -> (Boolean array=w258:bool[])
              n160 = Replace Array Subset(array=w258, new element=w255, index=6 ("索引")) -> (w256:bool[])
              n161 = Boolean Array To Number(Boolean array=w256) -> (number=w259:u32)
              n162 = To Unsigned Word Integer(number=w259) -> (unsigned 16bit integer=w254:u16)
              n163 = Build Array(w254) -> (w253:u16[])
              n164 = call "1553B_CMD.vi"("数据字数组"=w253) -> ("1553B指令"=w252:string)  [unwired: 10 in]
              n165 = in-place-cluster #14("主份控制指令"=w254, "信息帧.数据"=w252) -> (w250:T4)
            }
            n166 = call <vilib>:"Add State(s) to Queue__jki_lib_state_machine.vi"("State(s) in (\"\")"=w249, "State(s) at Back (\"\")"="Request:Write>>1553B_CMD_Zhufen") -> ("States Out"=w247:string)  [unwired: 13 in]
          }
          event "备份加计1加电": Value Change {
            n167 = event-data() -> ()  [unwired: 1 in, 6 out]
            n168 = in-place {
              in-place-border: bool[] [TRUE, FALSE] -> [w271]
              n169 = in-place-cluster #15(w267) -> ("主份控制指令"=w276:u16)  [unwired: 1 out]
              n170 = Number To Boolean Array(number=w276) -> (Boolean array=w274:bool[])
              n171 = Replace Array Subset(array=w274, new element=w271, index=6 ("索引")) -> (w272:bool[])
              n172 = Boolean Array To Number(Boolean array=w272) -> (number=w275:u32)
              n173 = To Unsigned Word Integer(number=w275) -> (unsigned 16bit integer=w270:u16)
              n174 = Build Array(w270) -> (w269:u16[])
              n175 = call "1553B_CMD.vi"("数据字数组"=w269) -> ("1553B指令"=w268:string)  [unwired: 10 in]
              n176 = in-place-cluster #15("主份控制指令"=w270, "信息帧.数据"=w268) -> (w266:T4)
            }
            n177 = call <vilib>:"Add State(s) to Queue__jki_lib_state_machine.vi"("State(s) in (\"\")"=w265, "State(s) at Back (\"\")"="Request:Write>>1553B_CMD_Beifen") -> ("States Out"=w263:string)  [unwired: 13 in]
          }
          event "备份加计1断电": Mouse Up {
            n178 = event-data() -> ()  [unwired: 1 in, 8 out]
            n179 = in-place {
              in-place-border: bool[] [FALSE, TRUE] -> [w287]
              n180 = in-place-cluster #16(w283) -> ("主份控制指令"=w292:u16)  [unwired: 1 out]
              n181 = Number To Boolean Array(number=w292) -> (Boolean array=w290:bool[])
              n182 = Replace Array Subset(array=w290, new element=w287, index=6 ("索引")) -> (w288:bool[])
              n183 = Boolean Array To Number(Boolean array=w288) -> (number=w291:u32)
              n184 = To Unsigned Word Integer(number=w291) -> (unsigned 16bit integer=w286:u16)
              n185 = Build Array(w286) -> (w285:u16[])
              n186 = call "1553B_CMD.vi"("数据字数组"=w285) -> ("1553B指令"=w284:string)  [unwired: 10 in]
              n187 = in-place-cluster #16("主份控制指令"=w286, "信息帧.数据"=w284) -> (w282:T4)
            }
            n188 = call <vilib>:"Add State(s) to Queue__jki_lib_state_machine.vi"("State(s) in (\"\")"=w281, "State(s) at Back (\"\")"="Request:Write>>1553B_CMD_Beifen") -> ("States Out"=w279:string)  [unwired: 13 in]
          }
          event "主份加计2加电": Value Change {
            n189 = event-data() -> ()  [unwired: 1 in, 6 out]
            n190 = in-place {
              in-place-border: bool[] [TRUE, FALSE] -> [w303]
              n191 = in-place-cluster #17(w299) -> ("主份控制指令"=w308:u16)  [unwired: 1 out]
              n192 = Number To Boolean Array(number=w308) -> (Boolean array=w306:bool[])
              n193 = Replace Array Subset(array=w306, new element=w303, index=8 ("索引")) -> (w304:bool[])
              n194 = Boolean Array To Number(Boolean array=w304) -> (number=w307:u32)
              n195 = To Unsigned Word Integer(number=w307) -> (unsigned 16bit integer=w302:u16)
              n196 = Build Array(w302) -> (w301:u16[])
              n197 = call "1553B_CMD.vi"("数据字数组"=w301) -> ("1553B指令"=w300:string)  [unwired: 10 in]
              n198 = in-place-cluster #17("主份控制指令"=w302, "信息帧.数据"=w300) -> (w298:T4)
            }
            n199 = call <vilib>:"Add State(s) to Queue__jki_lib_state_machine.vi"("State(s) in (\"\")"=w297, "State(s) at Back (\"\")"="Request:Write>>1553B_CMD_Zhufen") -> ("States Out"=w295:string)  [unwired: 13 in]
          }
          event "主份加计2断电": Mouse Up {
            n200 = event-data() -> ()  [unwired: 1 in, 8 out]
            n201 = in-place {
              in-place-border: bool[] [FALSE, TRUE] -> [w319]
              n202 = in-place-cluster #18(w315) -> ("主份控制指令"=w324:u16)  [unwired: 1 out]
              n203 = Number To Boolean Array(number=w324) -> (Boolean array=w322:bool[])
              n204 = Replace Array Subset(array=w322, new element=w319, index=8 ("索引")) -> (w320:bool[])
              n205 = Boolean Array To Number(Boolean array=w320) -> (number=w323:u32)
              n206 = To Unsigned Word Integer(number=w323) -> (unsigned 16bit integer=w318:u16)
              n207 = Build Array(w318) -> (w317:u16[])
              n208 = call "1553B_CMD.vi"("数据字数组"=w317) -> ("1553B指令"=w316:string)  [unwired: 10 in]
              n209 = in-place-cluster #18("主份控制指令"=w318, "信息帧.数据"=w316) -> (w314:T4)
            }
            n210 = call <vilib>:"Add State(s) to Queue__jki_lib_state_machine.vi"("State(s) in (\"\")"=w313, "State(s) at Back (\"\")"="Request:Write>>1553B_CMD_Zhufen") -> ("States Out"=w311:string)  [unwired: 13 in]
          }
          event "备份加计2加电": Value Change {
            n211 = event-data() -> ()  [unwired: 1 in, 6 out]
            n212 = in-place {
              in-place-border: bool[] [TRUE, FALSE] -> [w335]
              n213 = in-place-cluster #19(w331) -> ("主份控制指令"=w340:u16)  [unwired: 1 out]
              n214 = Number To Boolean Array(number=w340) -> (Boolean array=w338:bool[])
              n215 = Replace Array Subset(array=w338, new element=w335, index=8 ("索引")) -> (w336:bool[])
              n216 = Boolean Array To Number(Boolean array=w336) -> (number=w339:u32)
              n217 = To Unsigned Word Integer(number=w339) -> (unsigned 16bit integer=w334:u16)
              n218 = Build Array(w334) -> (w333:u16[])
              n219 = call "1553B_CMD.vi"("数据字数组"=w333) -> ("1553B指令"=w332:string)  [unwired: 10 in]
              n220 = in-place-cluster #19("主份控制指令"=w334, "信息帧.数据"=w332) -> (w330:T4)
            }
            n221 = call <vilib>:"Add State(s) to Queue__jki_lib_state_machine.vi"("State(s) in (\"\")"=w329, "State(s) at Back (\"\")"="Request:Write>>1553B_CMD_Beifen") -> ("States Out"=w327:string)  [unwired: 13 in]
          }
          event "备份加计2断电": Mouse Up {
            n222 = event-data() -> ()  [unwired: 1 in, 8 out]
            n223 = in-place {
              in-place-border: bool[] [FALSE, TRUE] -> [w351]
              n224 = in-place-cluster #20(w347) -> ("主份控制指令"=w356:u16)  [unwired: 1 out]
              n225 = Number To Boolean Array(number=w356) -> (Boolean array=w354:bool[])
              n226 = Replace Array Subset(array=w354, new element=w351, index=8 ("索引")) -> (w352:bool[])
              n227 = Boolean Array To Number(Boolean array=w352) -> (number=w355:u32)
              n228 = To Unsigned Word Integer(number=w355) -> (unsigned 16bit integer=w350:u16)
              n229 = Build Array(w350) -> (w349:u16[])
              n230 = call "1553B_CMD.vi"("数据字数组"=w349) -> ("1553B指令"=w348:string)  [unwired: 10 in]
              n231 = in-place-cluster #20("主份控制指令"=w350, "信息帧.数据"=w348) -> (w346:T4)
            }
            n232 = call <vilib>:"Add State(s) to Queue__jki_lib_state_machine.vi"("State(s) in (\"\")"=w345, "State(s) at Back (\"\")"="Request:Write>>1553B_CMD_Beifen") -> ("States Out"=w343:string)  [unwired: 13 in]
          }
          event "主份加计3加电": Value Change {
            n233 = event-data() -> ()  [unwired: 1 in, 6 out]
            n234 = in-place {
              in-place-border: bool[] [TRUE, FALSE] -> [w367]
              n235 = in-place-cluster #21(w363) -> ("主份控制指令"=w372:u16)  [unwired: 1 out]
              n236 = Number To Boolean Array(number=w372) -> (Boolean array=w370:bool[])
              n237 = Replace Array Subset(array=w370, new element=w367, index=10 ("索引")) -> (w368:bool[])
              n238 = Boolean Array To Number(Boolean array=w368) -> (number=w371:u32)
              n239 = To Unsigned Word Integer(number=w371) -> (unsigned 16bit integer=w366:u16)
              n240 = Build Array(w366) -> (w365:u16[])
              n241 = call "1553B_CMD.vi"("数据字数组"=w365) -> ("1553B指令"=w364:string)  [unwired: 10 in]
              n242 = in-place-cluster #21("主份控制指令"=w366, "信息帧.数据"=w364) -> (w362:T4)
            }
            n243 = call <vilib>:"Add State(s) to Queue__jki_lib_state_machine.vi"("State(s) in (\"\")"=w361, "State(s) at Back (\"\")"="Request:Write>>1553B_CMD_Zhufen") -> ("States Out"=w359:string)  [unwired: 13 in]
          }
          event "主份加计3断电": Mouse Up {
            n244 = event-data() -> ()  [unwired: 1 in, 8 out]
            n245 = in-place {
              in-place-border: bool[] [FALSE, TRUE] -> [w383]
              n246 = in-place-cluster #22(w379) -> ("主份控制指令"=w388:u16)  [unwired: 1 out]
              n247 = Number To Boolean Array(number=w388) -> (Boolean array=w386:bool[])
              n248 = Replace Array Subset(array=w386, new element=w383, index=10 ("索引")) -> (w384:bool[])
              n249 = Boolean Array To Number(Boolean array=w384) -> (number=w387:u32)
              n250 = To Unsigned Word Integer(number=w387) -> (unsigned 16bit integer=w382:u16)
              n251 = Build Array(w382) -> (w381:u16[])
              n252 = call "1553B_CMD.vi"("数据字数组"=w381) -> ("1553B指令"=w380:string)  [unwired: 10 in]
              n253 = in-place-cluster #22("主份控制指令"=w382, "信息帧.数据"=w380) -> (w378:T4)
            }
            n254 = call <vilib>:"Add State(s) to Queue__jki_lib_state_machine.vi"("State(s) in (\"\")"=w377, "State(s) at Back (\"\")"="Request:Write>>1553B_CMD_Zhufen") -> ("States Out"=w375:string)  [unwired: 13 in]
          }
          event "备份加计3加电": Value Change {
            n255 = event-data() -> ()  [unwired: 1 in, 6 out]
            n256 = in-place {
              in-place-border: bool[] [TRUE, FALSE] -> [w399]
              n257 = in-place-cluster #23(w395) -> ("主份控制指令"=w404:u16)  [unwired: 1 out]
              n258 = Number To Boolean Array(number=w404) -> (Boolean array=w402:bool[])
              n259 = Replace Array Subset(array=w402, new element=w399, index=10 ("索引")) -> (w400:bool[])
              n260 = Boolean Array To Number(Boolean array=w400) -> (number=w403:u32)
              n261 = To Unsigned Word Integer(number=w403) -> (unsigned 16bit integer=w398:u16)
              n262 = Build Array(w398) -> (w397:u16[])
              n263 = call "1553B_CMD.vi"("数据字数组"=w397) -> ("1553B指令"=w396:string)  [unwired: 10 in]
              n264 = in-place-cluster #23("主份控制指令"=w398, "信息帧.数据"=w396) -> (w394:T4)
            }
            n265 = call <vilib>:"Add State(s) to Queue__jki_lib_state_machine.vi"("State(s) in (\"\")"=w393, "State(s) at Back (\"\")"="Request:Write>>1553B_CMD_Beifen") -> ("States Out"=w391:string)  [unwired: 13 in]
          }
          event "备份加计3断电": Mouse Up {
            n266 = event-data() -> ()  [unwired: 1 in, 8 out]
            n267 = in-place {
              in-place-border: bool[] [FALSE, TRUE] -> [w415]
              n268 = in-place-cluster #24(w411) -> ("主份控制指令"=w420:u16)  [unwired: 1 out]
              n269 = Number To Boolean Array(number=w420) -> (Boolean array=w418:bool[])
              n270 = Replace Array Subset(array=w418, new element=w415, index=10 ("索引")) -> (w416:bool[])
              n271 = Boolean Array To Number(Boolean array=w416) -> (number=w419:u32)
              n272 = To Unsigned Word Integer(number=w419) -> (unsigned 16bit integer=w414:u16)
              n273 = Build Array(w414) -> (w413:u16[])
              n274 = call "1553B_CMD.vi"("数据字数组"=w413) -> ("1553B指令"=w412:string)  [unwired: 10 in]
              n275 = in-place-cluster #24("主份控制指令"=w414, "信息帧.数据"=w412) -> (w410:T4)
            }
            n276 = call <vilib>:"Add State(s) to Queue__jki_lib_state_machine.vi"("State(s) in (\"\")"=w409, "State(s) at Back (\"\")"="Request:Write>>1553B_CMD_Beifen") -> ("States Out"=w407:string)  [unwired: 13 in]
          }
          event "主份复位": Value Change {
            n277 = event-data() -> ("NewVal"=w423:bool)  [unwired: 1 in, 5 out]
            n278 = Select(t=bool[] [TRUE, FALSE], s=w423, f=bool[] [FALSE, TRUE]) -> (s? t:f=w424:bool[])
            n279 = call <vilib>:"Add State(s) to Queue__jki_lib_state_machine.vi"("State(s) in (\"\")"=w430, "State(s) at Back (\"\")"="Request:Write>>1553B_CMD_Zhufen") -> ("States Out"=w428:string)  [unwired: 13 in]
            n280 = in-place {
              in-place-border: w424 -> [w434]
              n281 = in-place-cluster #25(w422) -> ("主份控制指令"=w439:u16)  [unwired: 1 out]
              n282 = Number To Boolean Array(number=w439) -> (Boolean array=w437:bool[])
              n283 = Replace Array Subset(array=w437, new element=w434, index=12 ("索引")) -> (w435:bool[])
              n284 = Boolean Array To Number(Boolean array=w435) -> (number=w438:u32)
              n285 = To Unsigned Word Integer(number=w438) -> (unsigned 16bit integer=w433:u16)
              n286 = Build Array(w433) -> (w432:u16[])
              n287 = call "1553B_CMD.vi"("数据字数组"=w432) -> ("1553B指令"=w431:string)  [unwired: 10 in]
              n288 = in-place-cluster #25("主份控制指令"=w433, "信息帧.数据"=w431) -> (w421:T4)
            }
          }
          event "主份加计全加电": Value Change {
            (unwired) u16 15 ("RT地址(默认：10000)")
            n289 = event-data() -> ()  [unwired: 1 in, 6 out]
            n290 = call "1553B_CMD_v4.vi"("控制指令子地址(默认：11010"=u16 26, "数据字数组"=u16[] [33153]) -> ("1553B指令"=w440:string)  [unwired: 9 in]
            n291 = call <vilib>:"Add State(s) to Queue__jki_lib_state_machine.vi"("State(s) in (\"\")"=w446, "State(s) at Back (\"\")"="Request:Write>>1553B_CMD_Zhufen") -> ("States Out"=w444:string)  [unwired: 13 in]
            n292 = Bundle By Name(cluster=w448, "信息帧.数据"=w440) -> (w447:T4)
          }
          event "备份加计全加电": Value Change {
            (unwired) u16 15 ("RT地址(默认：10000)")
            n293 = event-data() -> ()  [unwired: 1 in, 6 out]
            n294 = call "1553B_CMD_v4.vi"("控制指令子地址(默认：11010"=u16 26, "数据字数组"=u16[] [33153]) -> ("1553B指令"=w449:string)  [unwired: 9 in]
            n295 = call <vilib>:"Add State(s) to Queue__jki_lib_state_machine.vi"("State(s) in (\"\")"=w455, "State(s) at Back (\"\")"="Request:Write>>1553B_CMD_Beifen") -> ("States Out"=w453:string)  [unwired: 13 in]
            n296 = Bundle By Name(cluster=w457, "信息帧.数据"=w449) -> (w456:T4)
          }
          event "主份加计全断电": Value Change {
            (unwired) u16 15 ("RT地址(默认：10000)")
            n297 = event-data() -> ()  [unwired: 1 in, 6 out]
            n298 = call "1553B_CMD_v4.vi"("控制指令子地址(默认：11010"=u16 26, "数据字数组"=u16[] [35466]) -> ("1553B指令"=w458:string)  [unwired: 9 in]
            n299 = call <vilib>:"Add State(s) to Queue__jki_lib_state_machine.vi"("State(s) in (\"\")"=w464, "State(s) at Back (\"\")"="Request:Write>>1553B_CMD_Zhufen") -> ("States Out"=w462:string)  [unwired: 13 in]
            n300 = Bundle By Name(cluster=w466, "信息帧.数据"=w458) -> (w465:T4)
          }
          event "备份加计全断电": Value Change {
            (unwired) u16 15 ("RT地址(默认：10000)")
            n301 = event-data() -> ()  [unwired: 1 in, 6 out]
            n302 = call "1553B_CMD_v4.vi"("控制指令子地址(默认：11010"=u16 26, "数据字数组"=u16[] [35466]) -> ("1553B指令"=w467:string)  [unwired: 9 in]
            n303 = call <vilib>:"Add State(s) to Queue__jki_lib_state_machine.vi"("State(s) in (\"\")"=w473, "State(s) at Back (\"\")"="Request:Write>>1553B_CMD_Beifen") -> ("States Out"=w471:string)  [unwired: 13 in]
            n304 = Bundle By Name(cluster=w475, "信息帧.数据"=w467) -> (w474:T4)
          }
          event "主份切大量程IF电路": Value Change {
            n305 = event-data() -> ()  [unwired: 1 in, 6 out]
            n306 = call "1553B_CMD_v4.vi"("控制指令子地址(默认：11010"=u16 26, "数据字数组"=u16[] [45489]) -> ("1553B指令"=w476:string)  [unwired: 9 in]
            n307 = call <vilib>:"Add State(s) to Queue__jki_lib_state_machine.vi"("State(s) in (\"\")"=w482, "State(s) at Back (\"\")"="Request:Write>>1553B_CMD_Zhufen") -> ("States Out"=w480:string)  [unwired: 13 in]
            n308 = Bundle By Name(cluster=w484, "信息帧.数据"=w476) -> (w483:T4)
          }
          event "备份切大量程IF电路": Value Change {
            n309 = event-data() -> ()  [unwired: 1 in, 6 out]
            n310 = call "1553B_CMD_v4.vi"("控制指令子地址(默认：11010"=u16 26, "数据字数组"=u16[] [45489]) -> ("1553B指令"=w485:string)  [unwired: 9 in]
            n311 = call <vilib>:"Add State(s) to Queue__jki_lib_state_machine.vi"("State(s) in (\"\")"=w491, "State(s) at Back (\"\")"="Request:Write>>1553B_CMD_Beifen") -> ("States Out"=w489:string)  [unwired: 13 in]
            n312 = Bundle By Name(cluster=w493, "信息帧.数据"=w485) -> (w492:T4)
          }
          event "主份切小量程IF电路": Value Change {
            (unwired) u16 15 ("RT地址(默认：10000)")
            n313 = event-data() -> ()  [unwired: 1 in, 6 out]
            n314 = call "1553B_CMD_v4.vi"("控制指令子地址(默认：11010"=u16 26, "数据字数组"=u16[] [47802]) -> ("1553B指令"=w494:string)  [unwired: 9 in]
            n315 = call <vilib>:"Add State(s) to Queue__jki_lib_state_machine.vi"("State(s) in (\"\")"=w500, "State(s) at Back (\"\")"="Request:Write>>1553B_CMD_Zhufen") -> ("States Out"=w498:string)  [unwired: 13 in]
            n316 = Bundle By Name(cluster=w502, "信息帧.数据"=w494) -> (w501:T4)
          }
          event "备份切小量程IF电路": Value Change {
            n317 = event-data() -> ()  [unwired: 1 in, 6 out]
            n318 = call "1553B_CMD_v4.vi"("控制指令子地址(默认：11010"=u16 26, "数据字数组"=u16[] [47802]) -> ("1553B指令"=w503:string)  [unwired: 9 in]
            n319 = call <vilib>:"Add State(s) to Queue__jki_lib_state_machine.vi"("State(s) in (\"\")"=w509, "State(s) at Back (\"\")"="Request:Write>>1553B_CMD_Beifen") -> ("States Out"=w507:string)  [unwired: 13 in]
            n320 = Bundle By Name(cluster=w511, "信息帧.数据"=w503) -> (w510:T4)
          }
          event "备份复位": Value Change {
            n321 = event-data() -> ("NewVal"=w512:bool)  [unwired: 1 in, 5 out]
            n322 = disable-structure shown="启用" {
              disable-tunnel: w518 -> [w523 w524]
              disable-tunnel: [w522 w525] -> w517
              disable-tunnel: w512 -> [_ w526]
              frame Disabled {
                n323 = call "1553B_CMD_v4.vi"("控制指令子地址(默认：11010"=u16 26, "数据字数组"=u16[] [10280]) -> ("1553B指令"=w519:string)  [unwired: 9 in]
                n324 = Bundle By Name(cluster=w523, "信息帧.数据"=w519) -> (w522:T4)
              }
              frame Enabled {
                n325 = Select(t=bool[] [TRUE], s=w526, f=bool[] [FALSE, TRUE]) -> (s? t:f=w527:bool[])
                n326 = in-place {
                  in-place-border: w527 -> [w533]
                  n327 = in-place-cluster #26(w524) -> ("主份控制指令"=w538:u16)  [unwired: 1 out]
                  n328 = Number To Boolean Array(number=w538) -> (Boolean array=w536:bool[])
                  n329 = Replace Array Subset(array=w536, new element=w533, index=12 ("索引")) -> (w534:bool[])
                  n330 = Boolean Array To Number(Boolean array=w534) -> (number=w537:u32)
                  n331 = To Unsigned Word Integer(number=w537) -> (unsigned 16bit integer=w532:u16)
                  n332 = Build Array(w532) -> (w531:u16[])
                  n333 = call "1553B_CMD.vi"("数据字数组"=w531) -> ("1553B指令"=w530:string)  [unwired: 10 in]
                  n334 = in-place-cluster #26("主份控制指令"=w532, "信息帧.数据"=w530) -> (w525:T4)
                }
              }
            }
            n335 = call <vilib>:"Add State(s) to Queue__jki_lib_state_machine.vi"("State(s) in (\"\")"=w516, "State(s) at Back (\"\")"="Request:Write>>1553B_CMD_Beifen") -> ("States Out"=w515:string)  [unwired: 13 in]
          }
          event "主份自定义周期": Value Change {
            n336 = event-data() -> ("NewVal"=w545:u16)  [unwired: 1 in, 5 out]
            n337 = property on="主份周期设置" class="RadioBtnsControl (严格)"() -> ("Value"=w540:enum32{"160ms", "自定义", "480ms", "10ms"})  [unwired: 2 in, 2 out]
            n338 = case shown="\"自定义\"" w540 {
              tunnel: w546 -> [w548 w554]
              tunnel: w545 -> [_ w549]
              tunnel: [w548 w553] -> w544
              tunnel: ["" "Config:Write>>1553B_CMD_Zhufen"] -> w539
              frame "160ms", Default {
              }
              frame "自定义" {
                n339 = Number To Decimal String(number=w549) -> (decimal integer string=w552:string)  [unwired: 1 in]
                n340 = Bundle By Name(cluster=w554, "信息帧.数据"=w552) -> (w553:T4)
                n341 = call <vilib>:"Write.vi"("Register name"="Zhufen_period", "Register value"=w549) -> ()  [unwired: 11 in, 3 out]
              }
            }
            n342 = call <vilib>:"Add State(s) to Queue__jki_lib_state_machine.vi"("State(s) in (\"\")"=w543, "State(s) at Back (\"\")"=w539) -> ("States Out"=w542:string)  [unwired: 13 in]
          }
          event "主份周期设置": Value Change {
            n343 = event-data() -> ("NewVal"=w561:enum32{"160ms", "自定义", "480ms", "10ms"})  [unwired: 1 in, 5 out]
            n344 = case shown="\"自定义\"" w561 {
              tunnel: [u16 160 ("Value") u16 10 ("Value") u16 480 ("Value") w575] -> w557
              tunnel: w559 -> [w567 w569 w571 w574]
              tunnel: [w567 w569 w571 w573] -> w556
              frame "160ms", Default {
              }
              frame "10ms" {
              }
              frame "480ms" {
              }
              frame "自定义" {
                n345 = property on="主份自定义周期" class="DigNum (严格)"(error in=w574) -> (error out=w573:errorcluster, "Value"=w575:u16)  [unwired: 1 in, 1 out]
              }
            }
            n346 = Number To Decimal String(number=w557) -> (decimal integer string=w560:string)  [unwired: 1 in]
            n347 = Bundle By Name(cluster=w566, "信息帧.数据"=w560) -> (w565:T4)
            n348 = call <vilib>:"Add State(s) to Queue__jki_lib_state_machine.vi"("State(s) in (\"\")"=w564, "State(s) at Back (\"\")"="Config:Write>>1553B_CMD_Zhufen") -> ("States Out"=w563:string)  [unwired: 13 in]
            n349 = call <vilib>:"Write.vi"("Register name"="Zhufen_period", "Register value"=w557, "Error in"=w556) -> ("Error out"=w555:errorcluster)  [unwired: 10 in, 2 out]
          }
          event "备份周期设置": Value Change {
            n350 = event-data() -> ("NewVal"=w578:enum32{"160ms", "自定义", "480ms", "10ms"})  [unwired: 1 in, 5 out]
            n351 = case shown="\"自定义\"" w578 {
              tunnel: [u16 160 ("Value") u16 10 ("Value") u16 480 ("Value") w596] -> w581
              tunnel: w579 -> [w588 w590 w592 w595]
              tunnel: [w588 w590 w592 w594] -> w580
              frame "160ms", Default {
              }
              frame "10ms" {
              }
              frame "480ms" {
              }
              frame "自定义" {
                n352 = property on="备份自定义周期" class="DigNum (严格)"(error in=w595) -> (error out=w594:errorcluster, "Value"=w596:u16)  [unwired: 1 in, 1 out]
              }
            }
            n353 = call <vilib>:"Add State(s) to Queue__jki_lib_state_machine.vi"("State(s) in (\"\")"=w585, "State(s) at Back (\"\")"="Config:Write>>1553B_CMD_Beifen") -> ("States Out"=w584:string)  [unwired: 13 in]
            n354 = Number To Decimal String(number=w581) -> (decimal integer string=w577:string)  [unwired: 1 in]
            n355 = Bundle By Name(cluster=w587, "信息帧.数据"=w577) -> (w586:T4)
            n356 = call <vilib>:"Write.vi"("Register name"="Beifen_period", "Register value"=w581, "Error in"=w580) -> ("Error out"=w576:errorcluster)  [unwired: 10 in, 2 out]
          }
          event "备份自定义周期": Value Change {
            n357 = event-data() -> ("NewVal"=w600:u16)  [unwired: 1 in, 5 out]
            n358 = property on="备份周期设置" class="RadioBtnsControl (严格)"(error in=w598) -> (error out=w597:errorcluster, "Value"=w599:enum32{"160ms", "自定义", "480ms", "10ms"})  [unwired: 1 in, 1 out]
            n359 = case shown="\"自定义\"" w599 {
              tunnel: w602 -> [w607 w612]
              tunnel: w600 -> [_ w611]
              tunnel: [w607 w610] -> w601
              tunnel: ["" "Config:Write>>1553B_CMD_Beifen"] -> w603
              frame "160ms", Default {
              }
              frame "自定义" {
                n360 = Number To Decimal String(number=w611) -> (decimal integer string=w609:string)  [unwired: 1 in]
                n361 = Bundle By Name(cluster=w612, "信息帧.数据"=w609) -> (w610:T4)
              }
            }
            n362 = call <vilib>:"Add State(s) to Queue__jki_lib_state_machine.vi"("State(s) in (\"\")"=w605, "State(s) at Back (\"\")"=w603) -> ("States Out"=w604:string)  [unwired: 13 in]
          }
          event "主份通道选择", "备份通道选择": Value Change {
            # "Request:OPEN1553B>>1553B_CMD_Zhufen\nRequest:OPEN1553B>>1553B_CMD_Beifen"
            n363 = event-data() -> ()  [unwired: 1 in, 6 out]
            n364 = in-place {
              n365 = in-place-cluster #27(w618) -> ()  [unwired: 1 out]
              n366 = Bundle By Name(cluster=T1 {"主份通道选择"=enum."通道A", "备份通道选择"=enum."通道B"} ("输入簇"), "主份通道选择"="主份通道选择", "备份通道选择"="备份通道选择") -> (w620:T1)
              n367 = Flatten To String(anything=w620) -> (data string=w619:string)  [unwired: 3 in, 2 out]
              n368 = in-place-cluster #27("信息帧.数据"=w619) -> (w617:T4)
            }
            n369 = call <vilib>:"Add State(s) to Queue__jki_lib_state_machine.vi"("State(s) in (\"\")"=w616, "State(s) at Back (\"\")"="Request:Write>>SwitchChanel\n") -> ("States Out"=w614:string)  [unwired: 13 in]
          }
          event "主份温控原状态", "主份温控关闭", "主份温控开启": Mouse Up {
            n370 = event-data() -> ("CtlRef"=w626:refnum<vi>)  [unwired: 1 in]
            n371 = property class="Bool (严格)"(reference=w626) -> ("Label.Text"=w625:string)  [unwired: 1 in, 2 out]
            n372 = case shown="\"主份温控原状态\", 默认" w625 {
              tunnel: [bool[] [TRUE, FALSE] bool[] [FALSE, TRUE] bool[] [TRUE, TRUE]] -> w624
              frame "主份温控开启" {
              }
              frame "主份温控关闭" {
              }
              frame "主份温控原状态", Default {
              }
            }
            n373 = in-place {
              in-place-border: w624 -> [w639]
              n374 = in-place-cluster #28(w632) -> ("主份控制指令"=w644:u16)  [unwired: 1 out]
              n375 = Number To Boolean Array(number=w644) -> (Boolean array=w642:bool[])
              n376 = Replace Array Subset(array=w642, new element=w639, index=14 ("索引")) -> (w640:bool[])
              n377 = Boolean Array To Number(Boolean array=w640) -> (number=w643:u32)
              n378 = To Unsigned Word Integer(number=w643) -> (unsigned 16bit integer=w638:u16)
              n379 = Build Array(w638) -> (w637:u16[])
              n380 = call "1553B_CMD.vi"("数据字数组"=w637) -> ("1553B指令"=w636:string)  [unwired: 10 in]
              n381 = in-place-cluster #28("主份控制指令"=w638, "信息帧.数据"=w636) -> (w631:T4)
            }
            n382 = call <vilib>:"Add State(s) to Queue__jki_lib_state_machine.vi"("State(s) in (\"\")"=w630, "State(s) at Back (\"\")"="Request:Write>>1553B_CMD_Zhufen") -> ("States Out"=w628:string)  [unwired: 13 in]
          }
          event "备份温控开启", "备份温控原状态", "备份温控关闭": Mouse Up {
            n383 = event-data() -> ("CtlRef"=w646:refnum<vi>)  [unwired: 1 in]
            n384 = property class="Bool (严格)"(reference=w646) -> ("Label.Text"=w647:string)  [unwired: 1 in, 2 out]
            n385 = case shown="\"备份温控原状态\", 默认" w647 {
              tunnel: [bool[] [TRUE, FALSE] bool[] [FALSE, TRUE] bool[] [TRUE, TRUE]] -> w645
              frame "备份温控开启" {
              }
              frame "备份温控关闭" {
              }
              frame "备份温控原状态", Default {
              }
            }
            n386 = in-place {
              in-place-border: w645 -> [w660]
              n387 = in-place-cluster #29(w653) -> ("主份控制指令"=w665:u16)  [unwired: 1 out]
              n388 = Number To Boolean Array(number=w665) -> (Boolean array=w663:bool[])
              n389 = Replace Array Subset(array=w663, new element=w660, index=14 ("索引")) -> (w661:bool[])
              n390 = Boolean Array To Number(Boolean array=w661) -> (number=w664:u32)
              n391 = To Unsigned Word Integer(number=w664) -> (unsigned 16bit integer=w659:u16)
              n392 = Build Array(w659) -> (w658:u16[])
              n393 = call "1553B_CMD.vi"("数据字数组"=w658) -> ("1553B指令"=w657:string)  [unwired: 10 in]
              n394 = in-place-cluster #29("主份控制指令"=w659, "信息帧.数据"=w657) -> (w652:T4)
            }
            n395 = call <vilib>:"Add State(s) to Queue__jki_lib_state_machine.vi"("State(s) in (\"\")"=w651, "State(s) at Back (\"\")"="Request:Write>>1553B_CMD_Beifen") -> ("States Out"=w649:string)  [unwired: 13 in]
          }
          event "主份复位远程终端": Value Change {
            n396 = event-data() -> ()  [unwired: 1 in, 6 out]
            n397 = in-place {
              n398 = in-place-cluster #30(w671) -> ()  [unwired: 1 out]
              n399 = call "1553B_Mode.vi"("模式命令"=u16 8, "RT地址"=u16 16) -> ("1553B指令"=w672:string)  [unwired: 9 in]
              n400 = in-place-cluster #30("信息帧.数据"=w672) -> (w670:T4)
            }
            n401 = call <vilib>:"Add State(s) to Queue__jki_lib_state_machine.vi"("State(s) in (\"\")"=w669, "State(s) at Back (\"\")"="Request:Write>>1553B_CMD_Zhufen") -> ("States Out"=w667:string)  [unwired: 13 in]
          }
          event "备份复位远程终端": Value Change {
            n402 = event-data() -> ()  [unwired: 1 in, 6 out]
            n403 = in-place {
              n404 = in-place-cluster #31(w680) -> ()  [unwired: 1 out]
              n405 = call "1553B_Mode.vi"("模式命令"=u16 8, "RT地址"=u16 16) -> ("1553B指令"=w681:string)  [unwired: 9 in]
              n406 = in-place-cluster #31("信息帧.数据"=w681) -> (w679:T4)
            }
            n407 = call <vilib>:"Add State(s) to Queue__jki_lib_state_machine.vi"("State(s) in (\"\")"=w678, "State(s) at Back (\"\")"="Request:Write>>1553B_CMD_Beifen") -> ("States Out"=w676:string)  [unwired: 13 in]
          }
          event "主份发送器关闭": Value Change {
            n408 = event-data() -> ()  [unwired: 1 in, 6 out]
            n409 = in-place {
              n410 = in-place-cluster #32(w689) -> ()  [unwired: 1 out]
              n411 = call "1553B_Mode.vi"("模式命令"=u16 4, "RT地址"=u16 16) -> ("1553B指令"=w690:string)  [unwired: 9 in]
              n412 = in-place-cluster #32("信息帧.数据"=w690) -> (w688:T4)
            }
            n413 = call <vilib>:"Add State(s) to Queue__jki_lib_state_machine.vi"("State(s) in (\"\")"=w687, "State(s) at Back (\"\")"="Request:Write>>1553B_CMD_Zhufen") -> ("States Out"=w685:string)  [unwired: 13 in]
          }
          event "备份发送器关闭": Value Change {
            n414 = event-data() -> ()  [unwired: 1 in, 6 out]
            n415 = in-place {
              n416 = in-place-cluster #33(w698) -> ()  [unwired: 1 out]
              n417 = call "1553B_Mode.vi"("模式命令"=u16 4, "RT地址"=u16 16) -> ("1553B指令"=w699:string)  [unwired: 9 in]
              n418 = in-place-cluster #33("信息帧.数据"=w699) -> (w697:T4)
            }
            n419 = call <vilib>:"Add State(s) to Queue__jki_lib_state_machine.vi"("State(s) in (\"\")"=w696, "State(s) at Back (\"\")"="Request:Write>>1553B_CMD_Beifen") -> ("States Out"=w694:string)  [unwired: 13 in]
          }
          event "主份取消发送器关闭": Value Change {
            n420 = event-data() -> ()  [unwired: 1 in, 6 out]
            n421 = in-place {
              n422 = in-place-cluster #34(w707) -> ()  [unwired: 1 out]
              n423 = call "1553B_Mode.vi"("模式命令"=u16 5, "RT地址"=u16 16) -> ("1553B指令"=w708:string)  [unwired: 9 in]
              n424 = in-place-cluster #34("信息帧.数据"=w708) -> (w706:T4)
            }
            n425 = call <vilib>:"Add State(s) to Queue__jki_lib_state_machine.vi"("State(s) in (\"\")"=w705, "State(s) at Back (\"\")"="Request:Write>>1553B_CMD_Zhufen") -> ("States Out"=w703:string)  [unwired: 13 in]
          }
          event "备份取消发送器关闭": Value Change {
            n426 = event-data() -> ()  [unwired: 1 in, 6 out]
            n427 = in-place {
              n428 = in-place-cluster #35(w716) -> ()  [unwired: 1 out]
              n429 = call "1553B_Mode.vi"("模式命令"=u16 5, "RT地址"=u16 16) -> ("1553B指令"=w717:string)  [unwired: 9 in]
              n430 = in-place-cluster #35("信息帧.数据"=w717) -> (w715:T4)
            }
            n431 = call <vilib>:"Add State(s) to Queue__jki_lib_state_machine.vi"("State(s) in (\"\")"=w714, "State(s) at Back (\"\")"="Request:Write>>1553B_CMD_Beifen") -> ("States Out"=w712:string)  [unwired: 13 in]
          }
          event "主份发送上一状态字": Value Change {
            n432 = event-data() -> ()  [unwired: 1 in, 6 out]
            n433 = in-place {
              n434 = in-place-cluster #36(w725) -> ()  [unwired: 1 out]
              n435 = call "1553B_Mode.vi"("模式命令"=u16 2, "RT地址"=u16 16) -> ("1553B指令"=w726:string)  [unwired: 9 in]
              n436 = in-place-cluster #36("信息帧.数据"=w726) -> (w724:T4)
            }
            n437 = call <vilib>:"Add State(s) to Queue__jki_lib_state_machine.vi"("State(s) in (\"\")"=w723, "State(s) at Back (\"\")"="Request:Write>>1553B_CMD_Zhufen") -> ("States Out"=w721:string)  [unwired: 13 in]
          }
          event "备份发送上一状态字": Value Change {
            n438 = event-data() -> ()  [unwired: 1 in, 6 out]
            n439 = in-place {
              n440 = in-place-cluster #37(w734) -> ()  [unwired: 1 out]
              n441 = call "1553B_Mode.vi"("模式命令"=u16 2, "RT地址"=u16 16) -> ("1553B指令"=w735:string)  [unwired: 9 in]
              n442 = in-place-cluster #37("信息帧.数据"=w735) -> (w733:T4)
            }
            n443 = call <vilib>:"Add State(s) to Queue__jki_lib_state_machine.vi"("State(s) in (\"\")"=w732, "State(s) at Back (\"\")"="Request:Write>>1553B_CMD_Beifen") -> ("States Out"=w730:string)  [unwired: 13 in]
          }
        }
      }
      frame "---------- Core ----------" {
        # "Do not put any code in this frame.\n(it is a separator no-op)"
        n444 = call <vilib>:"Add State(s) to Queue__jki_lib_state_machine.vi"("State(s) in (\"\")"=w741) -> ("States Out"=w740:string)  [unwired: 14 in]
      }
      frame Default {
        w751 = 42 items=["No error", "Argument error", "Memory is full", "Out of zone", "End of file", "File already open", "Generic file I/O error", "File not found", "File permission error", "Disk is full", "Duplicate path", "Too many files open", "System feature not enabled", "Resource file not found", "Cannot add resource", "Resource not found", "Image not found", "Image memory error", "Pen does not exist", "Config type invalid", "Config token not found", "Config parse error", "Config memory error", "Bad external code format", "Bad external code offset", "External code not present", "Null window", "Destroy window error", "Null menu", "Print aborted", "Bad print record", "Print driver error", "Windows error during printing", "Memory error during printing", "Print dialog error", "Generic print error", "Invalid device refnum", "Device not found", "Device parameter error", "Device unit error", "Cannot open device", "Device call aborted", "Generic error", "Cancelled by user", "Object ID too low", "Object ID too high", "Object not in heap", "Unknown heap", "Unknown object (invalid DefProc)", "Unknown object (DefProc not in table)", "Message out of range", "Invalid (null) method", "Unknown message", "Manager call not supported", "Bad address", "Network operation in progress", "Network operation timed out", "Connection is busy", "Network attribute not supported", "Network error", "Address in use", "System out of memory", "Connection aborted", "Connection refused", "Not connected", "Already connected", "Connection closed", "Initialization error (interapplication manager)", "Bad occurrence", "Wait on unbound occurrence handler", "Occurrence queue overflow", "Datalog type conflict", "Unused", "Unrecognized type (interapplication manager)", "Memory corrupt", "Failed to make temporary DLL", "Old CIN version", "Drag socket not found", "Failed to load drop-object", "Failed to register OLE object", "Failed to release OLE object", "Format specifier type mismatch", "Unknown format specifier", "Too few format specifiers", "Too many format specifiers", "Scan failed", "Newer CIN version", "Error converting to variant", "Runtime menu error", "Password tampered", "Variant attribute not found", "Incompatible variant data type", "Event data is not available", "Event Store is not present", "Occurrence is not found", "Event Queue is not created", "Event info is not available", "Refnum passed is NULL", "Error retrieving Class GUID", "Error retrieving CoClass GUID", "Error retrieving TypeLib GUID.", "Bad built application magic bytes.", "Specific driver is different from the specific driver associated with the Logical Name.", "There is no session opened to the class driver.", "Max Error", "MAX - Error with config objects", "MAX - Error loading configuration", "MAX - Group not supported"]
        # "Current State"
        # "Do not delete, rename, or modify this frame.\n(this is used to capture unhandled states and typos)"
        # "Handle mistyped state name (developer tool)"
        n445 = Format Into String(format string="Software Exception: Unhandled State \"%s\"." ("message"), error in=w747, w742) -> (resulting string=w750:string, error out=w749:errorcluster)  [unwired: 1 in]
        n446 = call <vilib>:"Error Cluster From Error Code.vi"("show call chain? (False)"=TRUE, "error in (no error)"=w749, "error message (\"\")"=w750, "error code (0)"=w751) -> ("error out"=w748:errorcluster)  [unwired: 5 in]
        n447 = call <vilib>:"Add State(s) to Queue__jki_lib_state_machine.vi"("State(s) in (\"\")"=w746) -> ("States Out"=w745:string)  [unwired: 14 in]
      }
      frame "Initialize Core Data" {
        # "Do not delete, rename, or modify this frame.\n(this is used to determine panel behavior on exit)"
        # "originally closed?"
        # "exe?"
        # "If panel starts closed or is an EXE, then close it when we exit"
        n448 = property class="VI"() -> ("Front Panel.Open"=w760:bool)  [unwired: 2 in, 2 out]
        n449 = property class="App"() -> ("App.Kind"=w759:T2)  [unwired: 2 in, 2 out]
        n450 = control-ref of="Current VI Reference"() -> (w753:refnum<vi>)
        n451 = Not(x=w760) -> (.not. x?=w757:bool)
        n452 = Equal?(x=w759, y=T2."Run Time System" ("Application:Kind")) -> (x = y?=w756:bool)
        n453 = Or(x=w757, y=w756) -> (x .or. y?=w754:bool)
        n454 = Bundle By Name(cluster=w755, "Core.Current VI Reference"=w753, "Core.Close Panel on Exit?"=w754) -> (w762:T4)
        n455 = call <vilib>:"Add State(s) to Queue__jki_lib_state_machine.vi"("State(s) in (\"\")"=w764) -> ("States Out"=w763:string)  [unwired: 14 in]
      }
      frame "Error Handler" {
        # "Unhandled Error -- Display it"
        # "Handle any errors here.\nYou can also output any states to clean-up after errors occur"
        # "Clear error"
        n456 = call <vilib>:"General Error Handler.vi"("error in (no error)"=w766) -> ()  [unwired: 10 in, 5 out]
        n457 = call <vilib>:"Add State(s) to Queue__jki_lib_state_machine.vi"("State(s) in Front (\"\")"="/* Post Error States", "State(s) in (\"\")"=w770) -> ("States Out"=w769:string)  [unwired: 13 in]
      }
      frame "Exit" {
        n458 = call <vilib>:"Add State(s) to Queue__jki_lib_state_machine.vi"("State(s) in (\"\")"=w775) -> ("States Out"=w774:string)  [unwired: 14 in]
      }
      frame "---------- Data ----------" {
        # "Do not put any code in this frame.\n(It is a separator no-op. You can make a copy of this frame to create a new Data frame)"
        n459 = call <vilib>:"Add State(s) to Queue__jki_lib_state_machine.vi"("State(s) in (\"\")"=w779) -> ("States Out"=w778:string)  [unwired: 14 in]
      }
      frame "Data: Initialize" {
        (unwired) enum32{"小量程", "大量程"}."小量程" ("加计大小量程")
        w780 = FALSE  # 定时控制
        w781 = i64 0  # 起始时间
        w782 = i64 0  # 秒计数
        w784 = u16 255  # 备份控制指令
        w785 = u16 255  # 主份控制指令
        w787 = T5 {" 数据帧名称"="", " 数据"="", "备用操作符"=TRUE, "起始地址"=0, "读写标志"=0, "长度"=0}  # 信息帧
        w788 = T6 {"Current VI Reference"=refnum, "Close Panel on Exit?"=FALSE}  # Core
        n460 = Bundle("Core"=w788, "传递队列输入"=w786, "信息帧"=w787, "主份控制指令"=w785, "备份控制指令"=w784, "notifier"=w783, "秒计数"=w782, "起始时间"=w781, "定时控制"=w780) -> (w790:T4)  [unwired: 1 in]
        n461 = call <vilib>:"Add State(s) to Queue__jki_lib_state_machine.vi"("State(s) in (\"\")"=w792) -> ("States Out"=w791:string)  [unwired: 14 in]
      }
      frame "Data: Cleanup" {
        # "Cleanup any data and references, here.\n(this is called automatically, by the Macro: Exit)"
        n462 = Unbundle By Name(w793) -> ("Core.Current VI Reference"=w796:refnum<vi>)
        n463 = Close Reference(reference=w796, error in (no error)=w795) -> (error out=w794:errorcluster)
        n464 = call <vilib>:"Add State(s) to Queue__jki_lib_state_machine.vi"("State(s) in (\"\")"=w798) -> ("States Out"=w797:string)  [unwired: 14 in]
      }
      frame "---------- UI ----------" {
        # "Do not put any code in this frame.\n(It is a separator no-op. You can make a copy of this frame to create a new UI frame)"
        n465 = call <vilib>:"Add State(s) to Queue__jki_lib_state_machine.vi"("State(s) in (\"\")"=w802) -> ("States Out"=w801:string)  [unwired: 14 in]
      }
      frame "UI: Initialize" {
        # "Initialize the User Interface, here.\n(this is called automatically, by the Macro: Init)"
        n466 = property on="主份周期设置" class="RadioBtnsControl (严格)"("Value"=enum32{"160ms", "自定义", "480ms", "10ms"}."10ms" ("主份周期设置")) -> ()  [unwired: 2 in, 2 out]
        n467 = property on="备份周期设置" class="RadioBtnsControl (严格)"("Value"=enum32{"160ms", "自定义", "480ms", "10ms"}."10ms" ("主份周期设置")) -> ()  [unwired: 2 in, 2 out]
        n468 = call <vilib>:"Add State(s) to Queue__jki_lib_state_machine.vi"("State(s) in (\"\")"=w808) -> ("States Out"=w807:string)  [unwired: 14 in]
      }
      frame "UI: Cursor Set" {
        # "Argument"
        # "Set and Unset Cursor Busy.\n(Usage: \"UI: Cursor Set >> Busy|Idle\")"
        n469 = case shown="\"Idle\", 默认" w809 {
          tunnel: w811 -> [w816 w818]
          tunnel: [w815 w817] -> w810
          frame "Idle", Default {
            n470 = call <vilib>:"Unset Busy.vi"("error in (no error)"=w816) -> ("error out"=w815:errorcluster)  [unwired: 10 in]
          }
          frame "Busy" {
            n471 = call <vilib>:"Set Busy.vi"("error in (no error)"=w818) -> ("error out"=w817:errorcluster)  [unwired: 9 in, 1 out]
          }
        }
        n472 = call <vilib>:"Add State(s) to Queue__jki_lib_state_machine.vi"("State(s) in (\"\")"=w814) -> ("States Out"=w813:string)  [unwired: 14 in]
      }
      frame "UI: Front Panel State" {
        # "Set Front Panel Open or Closed\n(Usage: \"UI: Front Panel State >> Open|Close\")"
        n473 = disable-structure shown="启用" {
          disable-tunnel: w822 -> [w829 w852]
          disable-tunnel: [w828 w852] -> w821
          disable-tunnel: w820 -> [w827 _]
          disable-tunnel: w819 -> [w825 _]
          frame Disabled {
            # "Argument"
            n474 = Unbundle By Name(w827) -> ("Core.Current VI Reference"=w826:refnum<vi>)
            n475 = case shown="\"Open\", 默认" w825 {
              tunnel: w829 -> [w833 w846]
              tunnel: [w835 w847] -> w828
              tunnel: w826 -> [w834 w844]
              frame "Open", Default {
                n476 = property class="VI"(reference=w834, error in=w833) -> (reference out=w831:refnum<vi>, error out=w832:errorcluster, "Front Panel.Open"=w830:bool)
                n477 = case shown="假" w830 {
                  tunnel: [w838 w841] -> w835
                  tunnel: w832 -> [w837 w841]
                  tunnel: w831 -> [w836 _]
                  frame False {
                    n478 = invoke class="VI" method="FP.Open"(reference=w836, error in=w837, "Activate"=TRUE, "State"=T3."Standard") -> (error out=w838:errorcluster)  [unwired: 1 in, 4 out]
                  }
                  frame True {
                  }
                }
              }
              frame "Close" {
                n479 = property class="VI"(reference=w844, error in=w846) -> (reference out=w843:refnum<vi>, error out=w845:errorcluster, "Front Panel.Open"=w842:bool)
                n480 = case shown="真" w842 {
                  tunnel: [w848 w851] -> w847
                  tunnel: w845 -> [w848 w850]
                  tunnel: w843 -> [_ w849]
                  frame False {
                  }
                  frame True {
                    n481 = invoke class="VI" method="FP.Close"(reference=w849, error in=w850) -> (error out=w851:errorcluster)  [unwired: 1 in, 2 out]
                  }
                }
              }
            }
          }
          frame Enabled {
          }
        }
        n482 = call <vilib>:"Add State(s) to Queue__jki_lib_state_machine.vi"("State(s) in (\"\")"=w824) -> ("States Out"=w823:string)  [unwired: 14 in]
      }
      frame "---------- Macro ----------" {
        # "Do not put any code in this frame.\n(It is a separator no-op. You can make a copy of this frame to create a new Macro frame)"
        n483 = call <vilib>:"Add State(s) to Queue__jki_lib_state_machine.vi"("State(s) in (\"\")"=w856) -> ("States Out"=w855:string)  [unwired: 14 in]
      }
      frame "Macro: Initialize" {
        w857 = "Data: Initialize\nInitialize Core Data\nUI: Initialize\nUI: Front Panel State >> Open"  # Data: Initialize Initialize Core Data UI: Initialize UI: Front Panel State >> Open
        # "Initialization Macro\n(This is called once, when the VI starts)"
        n484 = call <vilib>:"Add State(s) to Queue__jki_lib_state_machine.vi"("State(s) in Front (\"\")"=w857, "State(s) in (\"\")"=w861) -> ("States Out"=w860:string)  [unwired: 13 in]
      }
      frame "Macro: Exit" {
        # "Exit Macro\n(This is called once, when the VI exits)"
        n485 = Unbundle By Name(w868) -> ("Core.Close Panel on Exit?"=w867:bool)
        n486 = Select(t="UI: Front Panel State >> Close", s=w867, f="") -> (s? t:f=w864:string)
        n487 = call <vilib>:"Add State(s) to Queue__jki_lib_state_machine.vi"("State(s) in (\"\")"=w864, "State(s) at Back (\"\")"="Data: Cleanup\nExit") -> ("States Out"=w862:string)  [unwired: 13 in]
        n488 = call <vilib>:"Add State(s) to Queue__jki_lib_state_machine.vi"("State(s) in Front (\"\")"=w862, "State(s) in (\"\")"=w871) -> ("States Out"=w870:string)  [unwired: 13 in]
      }
      frame "----------Request----------" {
        # "Template Separator\n(You can make a copy of, or modify, this frame)"
        n489 = call <vilib>:"Add State(s) to Queue__jki_lib_state_machine.vi"("State(s) in (\"\")"=w875) -> ("States Out"=w874:string)  [unwired: 14 in]
      }
      frame "Request:Write" {
        n490 = in-place {
          in-place-border: w879 -> [w886]
          in-place-border: [w885] -> w878
          in-place-border: w876 -> [w884]
          n491 = in-place-cluster #38(w880) -> ("传递队列输入"=w890:refnum<queue>, "信息帧"=w889:T5)  [unwired: 1 out]
          n492 = in-place {
            in-place-border: w884 -> [w891]
            n493 = in-place-cluster #39(w889) -> ("数据"=w896:string)  [unwired: 5 out]
            n494 = in-place-cluster #39("数据帧名称"=w891, "数据"=w896, "备用操作符"=TRUE, "起始地址"=0, "读写标志"=1, "长度"=0) -> (w888:T5)
          }
          n495 = Enqueue Element(queue=w890, element=w888, error in (no error)=w886) -> (queue out=w887:refnum<queue>, error out=w885:errorcluster)  [unwired: 1 in, 1 out]
          n496 = in-place-cluster #38("传递队列输入"=w887, "信息帧"=w888, "主份控制指令"=u16 255) -> (w877:T4)
        }
        n497 = call <vilib>:"Add State(s) to Queue__jki_lib_state_machine.vi"("State(s) in (\"\")"=w882) -> ("States Out"=w881:string)  [unwired: 14 in]
      }
      frame "Config:Write" {
        n498 = in-place {
          in-place-border: w900 -> [w906]
          in-place-border: [w905] -> w899
          in-place-border: w897 -> [w904]
          n499 = in-place-cluster #40(w901) -> ("传递队列输入"=w910:refnum<queue>, "信息帧"=w909:T5)
          n500 = in-place {
            in-place-border: w904 -> [w911]
            n501 = in-place-cluster #41(w909) -> ("数据"=w916:string)  [unwired: 5 out]
            n502 = in-place-cluster #41("数据帧名称"=w911, "数据"=w916, "备用操作符"=TRUE, "起始地址"=0, "读写标志"=2, "长度"=0) -> (w908:T5)
          }
          n503 = Enqueue Element(queue=w910, element=w908, error in (no error)=w906) -> (queue out=w907:refnum<queue>, error out=w905:errorcluster)  [unwired: 1 in, 1 out]
          n504 = in-place-cluster #40("传递队列输入"=w907, "信息帧"=w908) -> (w898:T4)
        }
        n505 = call <vilib>:"Add State(s) to Queue__jki_lib_state_machine.vi"("State(s) in (\"\")"=w903) -> ("States Out"=w902:string)  [unwired: 14 in]
      }
      frame "Request:OPEN1553B" {
        n506 = in-place {
          in-place-border: w920 -> [w927]
          in-place-border: [w926] -> w919
          in-place-border: w917 -> [w924]
          n507 = in-place-cluster #42(w921) -> ("传递队列输入"=w930:refnum<queue>, "信息帧"=w925:T5)
          n508 = in-place {
            in-place-border: w924 -> [w931]
            n509 = in-place-cluster #43(w925) -> ()  [unwired: 6 out]
            n510 = in-place-cluster #43("数据帧名称"=w931, "数据"="$B\n", "备用操作符"=TRUE, "起始地址"=0, "读写标志"=1, "长度"=0) -> (w929:T5)
          }
          n511 = Enqueue Element(queue=w930, element=w929, error in (no error)=w927) -> (queue out=w928:refnum<queue>, error out=w926:errorcluster)  [unwired: 1 in, 1 out]
          n512 = in-place-cluster #42("传递队列输入"=w928, "信息帧"=w925) -> (w918:T4)
        }
        n513 = call <vilib>:"Add State(s) to Queue__jki_lib_state_machine.vi"("State(s) in (\"\")"=w923) -> ("States Out"=w922:string)  [unwired: 14 in]
      }
      frame "Request:Close1553B" {
        n514 = in-place {
          in-place-border: w939 -> [w948]
          in-place-border: [w947] -> w938
          n515 = in-place-cluster #44(w940) -> ("传递队列输入"=w950:refnum<queue>, "信息帧"=w944:T5)
          n516 = in-place {
            n517 = in-place-cluster #45(w944) -> ()  [unwired: 6 out]
            n518 = in-place-cluster #45("数据帧名称"="1553B_CMD", "数据"="$", "备用操作符"=TRUE, "起始地址"=0, "读写标志"=1, "长度"=0) -> (w949:T5)
          }
          n519 = in-place {
            n520 = in-place-cluster #46(w944) -> ()  [unwired: 6 out]
            n521 = in-place-cluster #46("数据帧名称"="1553B_CMD", "数据"="$Z\n", "备用操作符"=TRUE, "起始地址"=0, "读写标志"=1, "长度"=0) -> (w945:T5)
          }
          n522 = Enqueue Element(queue=w950, element=w949, error in (no error)=w948) -> (queue out=w946:refnum<queue>, error out=w947:errorcluster)  [unwired: 1 in, 1 out]
          n523 = Enqueue Element(queue=w946, element=w945) -> (queue out=w943:refnum<queue>)  [unwired: 2 in, 2 out]
          n524 = in-place-cluster #44("传递队列输入"=w943, "信息帧"=w944) -> (w937:T4)
        }
        n525 = call <vilib>:"Add State(s) to Queue__jki_lib_state_machine.vi"("State(s) in (\"\")"=w942) -> ("States Out"=w941:string)  [unwired: 14 in]
      }
      frame "Request:Read" {
        n526 = in-place {
          in-place-border: w965 -> [w970]
          in-place-border: [w969] -> w964
          n527 = in-place-cluster #47(w966) -> ("传递队列输入"=w974:refnum<queue>, "信息帧"=w973:T5)
          n528 = in-place {
            n529 = in-place-cluster #48(w973) -> ("数据"=w979:string)  [unwired: 5 out]
            n530 = in-place-cluster #48("数据帧名称"="GNSS1", "数据"=w979, "备用操作符"=TRUE, "起始地址"=0, "读写标志"=0, "长度"=0) -> (w972:T5)
          }
          n531 = Enqueue Element(queue=w974, element=w972, error in (no error)=w970) -> (queue out=w971:refnum<queue>, error out=w969:errorcluster)  [unwired: 1 in, 1 out]
          n532 = in-place-cluster #47("传递队列输入"=w971, "信息帧"=w972) -> (w963:T4)
        }
        n533 = call <vilib>:"Add State(s) to Queue__jki_lib_state_machine.vi"("State(s) in (\"\")"=w968) -> ("States Out"=w967:string)  [unwired: 14 in]
      }
      frame "----------Usr----------" {
        # "Template Separator\n(You can make a copy of, or modify, this frame)"
        n534 = call <vilib>:"Add State(s) to Queue__jki_lib_state_machine.vi"("State(s) in (\"\")"=w984) -> ("States Out"=w983:string)  [unwired: 14 in]
      }
      frame "Exit:all" {
        n535 = call <vilib>:"Add State(s) to Queue__jki_lib_state_machine.vi"("State(s) in Front (\"\")"="Macro: Exit", "State(s) in (\"\")"=w989) -> ("States Out"=w988:string)  [unwired: 13 in]
      }
    }
  }
  n536 = while {
    tunnel: "notifier" -> [w998]
    stop <- w997 stop-if-true
    n537 = call "stop_message.vi"("notifier"=w998) -> ("Exit？"=w997:bool)  [unwired: 9 in, 1 out]
    n538 = Wait Until Next ms Multiple(millisecond multiple=u32 200 ("毫秒倍数")) -> ()  [unwired: 1 out]
    n539 = call <vilib>:"Read.vi"("Register name"="AIs") -> ("Register value"=w995:variant)  [unwired: 11 in, 3 out]
    n540 = call-poly <vilib>:"Convert.vi"("Register value in"=w995) -> ("Register value out"=w994:sgl[])  [unwired: 13 in, 1 out]
    n541 = for {
      N: 9 -> [_]
      tunnel: w994 -> [w1006] mode=indexing
      shift-right: [w1007] -> w992
      shift-left: "模拟量\n\n" -> [w1000]
      tunnel: string[] ["外部模拟量", "A_LTU电源遥测", "B_LTU电源遥测", "G1陀螺电源遥测", "G2陀螺电源遥测", "G3陀螺电源遥测", "A1加计电源遥测", "A2加计电源遥测", "A3加计电源遥测"] -> [w1001] mode=indexing
      n542 = Concatenate Strings(w1001, "                     " ("字符串")) -> (w1004:string)
      n543 = String Subset(string=w1004, length (rest)=16 ("长度（剩余）")) -> (substring=w1002:string)  [unwired: 1 in]
      n544 = Number To Fractional String(number=w1006, width (-)=i16 6 ("宽度(-)"), precision (6)=i16 3 ("精度(6)")) -> (F-format string=w1009:string)  [unwired: 1 in]
      n545 = Concatenate Strings(w1000, w1002, w1009, "\n") -> (w1007:string)
    }
    "模拟量显示区" <- w992
  }
